vi "CRYRTA.vi"(0 "Device In":u16, 2 "Manual":bool=TRUE, 5 "Signal Path":i32(ring) caption="信号通道", 7 "Avg. Time(sec)":dbl=0.05 caption="平均时间(秒)" min=0.05 format="%.0p", 9 "Weighting":i32(ring) caption="加权" items=["Linear", "A-weighting", "B-weighting", "C-weighting", "ITU-R 468-4", "Dolby", "CCITT", "C-message", "Wb", "Wc", "Wd", "We", "Wf", "Wh", "Wj", "Wk", "Wm", "AES17 20 kHz lowpass", "AES17 40 kHz lowpass", "AES17 20 kHz highpass", "AES17 40 kHz highpass"], 11 "Start":bool, 12 "Hardware in":string, 13 "Execution control":T8={"interactive"=TRUE, "displayed"=TRUE, "in a seq"=FALSE}, 14 "Calibration in":string) -> (3 "Canceled?":bool, 4 "band power":dbl[](array[numeric]), 6 "Data output":T4, 8 "df Array":dbl[](array[numeric]), 10 "Data Out":T6={"Name"="", "Curve"=[], "X data"=1, "Y data"=1, "Z data"=1, "X axis"=0, "Y axis"=1, "Z axis"=1, "X unit"="", "Y unit"="", "Z unit"="", "X dB ref"=1.0, "Y dB ref"=1.0, "Z dB ref"=1.0, "single val"=FALSE, "protected"=FALSE, "display X"=TRUE, "display Y"=FALSE, "display Z"=TRUE, "Test Info"="", "Step No."=0, "Plot Settings"={"Color"=0, "Interpolation"=0, "Point Style"=0, "Line Style"=0, "Point Color"=0, "Line Width"=0, "Bar Plot Style"=0, "Fill To"=0}, "AutoProtect"=FALSE} {"Z data" items=["dB", "Lin"]; "X data" items=["dB", "Lin"]; "Y data" items=["dB", "Lin"]; "Z dB ref" format="%.1f"; "Z axis" items=["Log", "Lin"]; "X dB ref" format="%.1f"; "X axis" items=["Log", "Lin"]; "Y axis" items=["Log", "Lin"]; "Y dB ref" format="%.1f"; "Curve"."z" format="%.2f"; "Curve"."y" format="%.2f"; "Curve"."x" format="%.2f"}, 15 "RTA Setup Out":string)   [LabVIEW 2013]
uses:
  Typedef Control/CRYData Cluster.ctl
  Typedef Control/CRYData Variant Array.ctl
  <vilib>/addons/_NISVFA/_Shared subVIs/Controls/svc_Channel Info.ctl
  <vilib>/addons/_NISVFA/_Shared subVIs/Controls/svc_Engineering Units Text Ring.ctl
  <vilib>/addons/_NISVFA/_Shared subVIs/Controls/svc_Weighting Filter Text Ring.ctl
  Typedef Control/CRYHardware Channel Info.ctl
  <vilib>/addons/Sound and Vibration/svt_Calibration/SVL Scale Voltage to EU (1 Ch).vi
  <vilib>/addons/_NISVFA/_Shared subVIs/Common/svc_Set SV Channel Info.vi
  <vilib>/addons/_NISVFA/_Shared subVIs/Common/svc_Set SV Channel Info (variant).vi
  <vilib>/addons/_NISVFA/_Shared subVIs/Common/SVL Set dB Reference (variant).vi
  SubVI/CRYMisc vis settings global.vi
  Calibration/SubVI/CRYCal Global.vi
  CRYMainGlobal.vi
  Task Sequence/CRYProject Run Control Global.vi
  <vilib>/addons/Sound and Vibration/svt_Octave/SVT Fractional-octave Analysis (1 Ch).vi
  <vilib>/addons/_NISVFA/_Shared subVIs/Common/svc_Engineering Units to Unit Label.vi
  <vilib>/addons/_NISVFA/_Shared subVIs/Common/svc_Compute Scale Factor to Convert V to EU.vi
  <vilib>/addons/_NISVFA/_Shared subVIs/Common/svc_Set dB ref if Pascal.vi
  <vilib>/addons/_NISVFA/_Shared subVIs/Common/svc_Caller VI Returned in Error Source.vi
  <vilib>/addons/Sound and Vibration/svt_Octave/SoundVib_Octave.lvlib
  CRYSound.dll
  <vilib>/addons/Sound and Vibration/svt_Calibration/SoundVib_Calibration.lvlib
panel:
  out "cal factor":dbl
  in  "equal confidence level [dB]":dbl=1.0
  in  "channel info":T1={"sensor sensitivity [mV/EU]"=1000.0, "engineering units"=1, "dB reference [EU]"=1.0, "custom label"="EU", "weighting filter"=0, "pregain [dB]"=0.0} {"pregain [dB]" format="%.2f"; "weighting filter" items=["Linear", "A-weighting", "B-weighting", "C-weighting", "ITU-R 468-4", "Dolby", "CCITT", "C-message", "Wb", "Wc", "Wd", "We", "Wf", "Wh", "Wj", "Wk", "Wm", "AES17 20 kHz lowpass", "AES17 40 kHz lowpass", "AES17 20 kHz highpass", "AES17 40 kHz highpass"]; "dB reference [EU]" format="%^.1e"; "engineering units" items=["custom..."=0, "V"=1, "A"=21, "Pa"=2, "N"=20, "g"=3, "m/s^2"=4, "m/s"=5, "m"=6, "mm/s"=12, "mm"=13, "micron/s"=14, "micron"=15, "in/s^2"=7, "in/s"=8, "in"=9, "mil/s"=10, "mil"=11, "rad/s^2"=16, "rad/s"=17, "rad"=18, "deg/s^2"=26, "deg/s"=27, "deg"=28, "RPM"=22, "cycle/s^2"=23, "Hz"=24, "cycle"=25, "strain"=19]; "sensor sensitivity [mV/EU]" format="%.2f"}
  in  "dB ref. 2":dbl=20.0 format="%.2f"
  in  "Buf Cnt":i32
  in  "isMain":bool
  in  "Rcv Idx":u16
  in  "start_flg":u8
  out "Asio OCI":u32
  in  "ASIO_Inited":bool
  in  "Remain Data":i32[](array[numeric])
  in  "Device Name":string
  in  "Audio Driver":u16
  out "error out 2":errorcluster
  out "initialized array":i32[](array[numeric])
  in  "taskID":u32
  out "Load Test":bool
  out "Configure Data":string
  out "Set Configure":bool
  out "Signal Graph":bool caption="显示"
  out "Averaging":bool caption="平均"
  out "Spectrum1":bool caption="频谱"
  out "Input":bool caption="输入"
  out "Menu":bool=TRUE
  out "StateOut":bool=TRUE
  out "VI nID":i32
  out "Title nID":i32
  in  "delta_Y":dbl
  in  "delta_X":dbl format="%#.3p"
  in  "delta_str":string
  in  "Data In":T5
  in  "Cancel":bool
  in  "Save":bool
  in  "OK":bool
  out "AvgT":bool
  in  "Continue":bool
  in  "Time Weighting":i32(ring) caption="时间加权" items=["快", "慢", "自定义"]
  in  "Lin/Exp":i32(slide)
  in  "Octave Band":u16(ring) caption="倍频程" items=["1/1", "1/3", "1/6", "1/12", "1/24"]
  in  "Correct":bool caption="应用修正"
  in  "A/M/M":i32(slide)
  out "Real Time":u16(slide) caption="实时" scale=0.0..10.0
  out "Buffer":u16(slide) caption="缓冲器" scale=0.0..100.0
  out "Spectrum":T7(graph)={"nominal frequencies [Hz]"=[16.00000023841858, 20.0, 25.0, 31.500000953674316, 40.0, 50.0, 63.00000190734863, 80.0, 100.0, 125.0, 160.0000023841858, 200.0, 250.0, 315.00000953674316, 400.0, 500.0, 630.0000190734863, 800.0, 1000.0, 1250.0, 1600.000023841858, 2000.0, 2500.0, 3150.0000953674316, 4000.0, 5000.0, 6300.000190734863, 8000.0, 10000.0, 12500.0, 16000.00023841858, 20000.0, 25000.0, 31500.000953674316, 40000.0, 50000.0], "band power"=[-69.88905633271838, -74.01516494128754, -77.58719522671365, -75.73752952138173, -71.3505823520545, -71.81115871325046, -70.64913806002016, -71.74459815152325, -68.26393707572068, -69.54637847470994, -67.93028521843318, -67.11517882984813, -62.609020897016414, -59.9132266385828, -59.334469065938535, -58.93600195892711, -54.76273997651711, -40.68205149663691, -35.92796599129668, -52.708171896456896, -58.27685035662345, -61.23526661320974, -63.279755740002244, -64.8500026443712, -66.18360537650693, -67.37703351590173, -68.4921051421575, -69.5202741642352, -70.56777995681341, -71.50671705937012, -72.52145445138709, -73.39348059691609, -74.16354227965358, -74.79422393268355, -75.18526767722105, -75.16825214452263]}
  in  "分支常量\n（见即时帮助）":bool
  in  "Record delay (ms)":dbl=100.0 format="%.2f"
  out "Elapsed Time":dbl=0.1 caption="消耗时间" format="%#.3p"
  in  "close at end":bool
  out "avg count":i32 caption="Averages"
  in  "A-weights table":dbl[][](array[numeric])=[[0.00012901551291928683, 0.001463404113537998, 0.01066103097242493, 0.04899156950274862, 0.156669051402536, 0.37020550818873904, 0.689209635331696, 0.9999999947155233, 1.148185035046126, 1.118252632301628, 0.8802313561816225, 0.0, 0.0, 0.0, 0.0, 0.0, 0.0, 0.0, 0.0, 0.0, 0.0, 0.0, 0.0, 0.0, 0.0, 0.0, 0.0, 0.0, 0.0, 0.0, 0.0, 0.0, 0.0, 0.0, 0.0, 0.0, 0.0, 0.0, 0.0, 0.0, 0.0, 0.0, 0.0, 0.0, 0.0, 0.0, 0.0, 0.0, 0.0, 0.0, 0.0, 0.0, 0.0, 0.0, 0.0, 0.0, 0.0, 0.0, 0.0, 0.0, 0.0, 0.0, 0.0, 0.0, 0.0, 0.0, 0.0, 0.0, 0.0, 0.0, 0.0, 0.0, 0.0, 0.0, 0.0, 0.0, 0.0, 0.0, 0.0, 0.0, 0.0, 0.0, 0.0, 0.0, 0.0, 0.0, 0.0, 0.0, 0.0, 0.0, 0.0, 0.0, 0.0, 0.0, 0.0, 0.0, 0.0, 0.0, 0.0, 0.0, 0.0, 0.0, 0.0, 0.0, 0.0, 0.0, 0.0, 0.0, 0.0, 0.0, 0.0, 0.0, 0.0, 0.0, 0.0, 0.0, 0.0, 0.0, 0.0, 0.0, 0.0, 0.0, 0.0, 0.0, 0.0, 0.0, 0.0, 0.0, 0.0, 0.0, 0.0, 0.0, 0.0, 0.0, 0.0, 0.0, 0.0, 0.0, 0.0, 0.0, 0.0, 0.0, 0.0, 0.0, 0.0, 0.0, 0.0, 0.0, 0.0, 0.0, 0.0, 0.0, 0.0, 0.0, 0.0, 0.0, 0.0, 0.0, 0.0, 0.0, 0.0, 0.0, 0.0, 0.0, 0.0, 0.0, 0.0, 0.0, 0.0, 0.0, 0.0, 0.0, 0.0, 0.0, 0.0, 0.0, 0.0, 0.0, 0.0, 0.0, 0.0, 0.0, 0.0, 0.0, 0.0, 0.0, 0.0, 0.0, 0.0, 0.0, 0.0, 0.0, 0.0, 0.0, 0.0, 0.0, 0.0, 0.0, 0.0, 0.0, 0.0, 0.0, 0.0, 0.0, 0.0, 0.0, 0.0, 0.0, 0.0, 0.0, 0.0, 0.0, 0.0, 0.0, 0.0, 0.0, 0.0, 0.0, 0.0, 0.0, 0.0, 0.0, 0.0, 0.0, 0.0, 0.0, 0.0, 0.0, 0.0, 0.0, 0.0, 0.0, 0.0, 0.0, 0.0, 0.0, 0.0, 0.0, 0.0, 0.0, 0.0, 0.0, 0.0, 0.0, 0.0, 0.0, 0.0, 0.0, 0.0, 0.0, 0.0, 0.0, 0.0, 0.0, 0.0, 0.0, 0.0, 0.0, 0.0, 0.0, 0.0, 0.0, 0.0, 0.0, 0.0, 0.0, 0.0, 0.0, 0.0, 0.0, 0.0, 0.0, 0.0, 0.0, 0.0, 0.0], [5.399407495978195e-05, 0.00012901551291928683, 0.00030077593224389377, 0.0006779776875028787, 0.001463404113537998, 0.0030003304333084445, 0.00581621210485118, 0.01066103097242493, 0.018547914314881855, 0.030790110186524937, 0.04899156950274862, 0.0749323365877836, 0.11034238899050194, 0.156669051402536, 0.2149857926605078, 0.2860385580343268, 0.37020550818873904, 0.4671091612550431, 0.5748515933740767, 0.689209635331696, 0.8034638534410672, 0.9094994307304253, 0.9999999947155233, 1.0704410251961953, 1.1195518850512476, 1.148185035046126, 1.1575955360559005, 1.1480657780180865, 1.118252632301628, 1.0653659406851155, 0.9863557110490331, 0.8802313561816225, 0.7509021647928303, 0.6086168184785875, 0.4678834620808579, 0.0, 0.0, 0.0, 0.0, 0.0, 0.0, 0.0, 0.0, 0.0, 0.0, 0.0, 0.0, 0.0, 0.0, 0.0, 0.0, 0.0, 0.0, 0.0, 0.0, 0.0, 0.0, 0.0, 0.0, 0.0, 0.0, 0.0, 0.0, 0.0, 0.0, 0.0, 0.0, 0.0, 0.0, 0.0, 0.0, 0.0, 0.0, 0.0, 0.0, 0.0, 0.0, 0.0, 0.0, 0.0, 0.0, 0.0, 0.0, 0.0, 0.0, 0.0, 0.0, 0.0, 0.0, 0.0, 0.0, 0.0, 0.0, 0.0, 0.0, 0.0, 0.0, 0.0, 0.0, 0.0, 0.0, 0.0, 0.0, 0.0, 0.0, 0.0, 0.0, 0.0, 0.0, 0.0, 0.0, 0.0, 0.0, 0.0, 0.0, 0.0, 0.0, 0.0, 0.0, 0.0, 0.0, 0.0, 0.0, 0.0, 0.0, 0.0, 0.0, 0.0, 0.0, 0.0, 0.0, 0.0, 0.0, 0.0, 0.0, 0.0, 0.0, 0.0, 0.0, 0.0, 0.0, 0.0, 0.0, 0.0, 0.0, 0.0, 0.0, 0.0, 0.0, 0.0, 0.0, 0.0, 0.0, 0.0, 0.0, 0.0, 0.0, 0.0, 0.0, 0.0, 0.0, 0.0, 0.0, 0.0, 0.0, 0.0, 0.0, 0.0, 0.0, 0.0, 0.0, 0.0, 0.0, 0.0, 0.0, 0.0, 0.0, 0.0, 0.0, 0.0, 0.0, 0.0, 0.0, 0.0, 0.0, 0.0, 0.0, 0.0, 0.0, 0.0, 0.0, 0.0, 0.0, 0.0, 0.0, 0.0, 0.0, 0.0, 0.0, 0.0, 0.0, 0.0, 0.0, 0.0, 0.0, 0.0, 0.0, 0.0, 0.0, 0.0, 0.0, 0.0, 0.0, 0.0, 0.0, 0.0, 0.0, 0.0, 0.0, 0.0, 0.0, 0.0, 0.0, 0.0, 0.0, 0.0, 0.0, 0.0, 0.0, 0.0, 0.0, 0.0, 0.0, 0.0, 0.0, 0.0, 0.0, 0.0, 0.0, 0.0, 0.0, 0.0, 0.0, 0.0, 0.0, 0.0, 0.0, 0.0, 0.0, 0.0, 0.0, 0.0, 0.0, 0.0, 0.0, 0.0, 0.0, 0.0, 0.0, 0.0, 0.0, 0.0, 0.0, 0.0, 0.0, 0.0, 0.0, 0.0, 0.0, 0.0, 0.0, 0.0, 0.0, 0.0, 0.0, 0.0], [8.367843089077905e-05, 0.00012901551291928683, 0.000197701205238207, 0.00030077593224389377, 0.0004537558525726572, 0.0006779776875028787, 0.0010020521461877657, 0.001463404113537998, 0.0021097598133486134, 0.0030003304333084445, 0.0042071775532512646, 0.00581621210485118, 0.007928313709042484, 0.01066103097242493, 0.014149403982936655, 0.018547914314881855, 0.024030527738545613, 0.030790110186524937, 0.039036565356906174, 0.04899156950274862, 0.0608822293261807, 0.0749323365877836, 0.09135462337865059, 0.11034238899050194, 0.132065471964561, 0.156669051402536, 0.18427522223316958, 0.2149857926605078, 0.24888545563454106, 0.2860385580343268, 0.32648117357435763, 0.37020550818873904, 0.41713765756791077, 0.4671091612550431, 0.5198278741632266, 0.5748515933740767, 0.6315709380291434, 0.689209635331696, 0.7468467914771676, 0.8034638534410672, 0.8580134792451037, 0.9094994307304253, 0.9570545361539051, 0.9999999947155233, 1.037876206708114, 1.0704410251961953, 1.0976390517709886, 1.1195518850512476, 1.1363399019935716, 1.148185035046126, 1.1552411946705066, 1.1575955360559005, 1.1552417895398122, 1.1480657780180865, 1.1358434838302867, 1.118252632301628, 1.0948998942166022, 1.0653659406851155, 1.029270469199537, 0.9863557110490331, 0.9365833197371723, 0.8802313561816225, 0.817971279008174, 0.7509021647928303, 0.6805201645952638, 0.6086168184785875, 0.537116348933795, 0.4678834620808579, 0.4025421323855877, 0.3423424643096228, 0.0, 0.0, 0.0, 0.0, 0.0, 0.0, 0.0, 0.0, 0.0, 0.0, 0.0, 0.0, 0.0, 0.0, 0.0, 0.0, 0.0, 0.0, 0.0, 0.0, 0.0, 0.0, 0.0, 0.0, 0.0, 0.0, 0.0, 0.0, 0.0, 0.0, 0.0, 0.0, 0.0, 0.0, 0.0, 0.0, 0.0, 0.0, 0.0, 0.0, 0.0, 0.0, 0.0, 0.0, 0.0, 0.0, 0.0, 0.0, 0.0, 0.0, 0.0, 0.0, 0.0, 0.0, 0.0, 0.0, 0.0, 0.0, 0.0, 0.0, 0.0, 0.0, 0.0, 0.0, 0.0, 0.0, 0.0, 0.0, 0.0, 0.0, 0.0, 0.0, 0.0, 0.0, 0.0, 0.0, 0.0, 0.0, 0.0, 0.0, 0.0, 0.0, 0.0, 0.0, 0.0, 0.0, 0.0, 0.0, 0.0, 0.0, 0.0, 0.0, 0.0, 0.0, 0.0, 0.0, 0.0, 0.0, 0.0, 0.0, 0.0, 0.0, 0.0, 0.0, 0.0, 0.0, 0.0, 0.0, 0.0, 0.0, 0.0, 0.0, 0.0, 0.0, 0.0, 0.0, 0.0, 0.0, 0.0, 0.0, 0.0, 0.0, 0.0, 0.0, 0.0, 0.0, 0.0, 0.0, 0.0, 0.0, 0.0, 0.0, 0.0, 0.0, 0.0, 0.0, 0.0, 0.0, 0.0, 0.0, 0.0, 0.0, 0.0, 0.0, 0.0, 0.0, 0.0, 0.0, 0.0, 0.0, 0.0, 0.0, 0.0, 0.0, 0.0, 0.0, 0.0, 0.0, 0.0, 0.0, 0.0, 0.0, 0.0, 0.0, 0.0, 0.0, 0.0, 0.0, 0.0, 0.0, 0.0, 0.0, 0.0, 0.0, 0.0, 0.0, 0.0, 0.0, 0.0, 0.0, 0.0, 0.0, 0.0, 0.0, 0.0, 0.0, 0.0, 0.0, 0.0, 0.0, 0.0, 0.0, 0.0, 0.0, 0.0, 0.0, 0.0, 0.0, 0.0, 0.0, 0.0, 0.0, 0.0, 0.0, 0.0, 0.0], [0.00011583993672799015, 0.0001436292864864441, 0.0001778012603656263, 0.00021973037298173516, 0.00027102570238892744, 0.00033361829503177585, 0.00040977096445946406, 0.000502144096454577, 0.0006138152751182365, 0.0007483329340285107, 0.0009097805203891802, 0.0011028293999198581, 0.0013327910595308504, 0.0016055412855545807, 0.001927812596850252, 0.0023069345626637503, 0.0027510762632911817, 0.0032692688858618688, 0.0038713529606718092, 0.004568038488373186, 0.005370988330067639, 0.00629273027705919, 0.007347006248508048, 0.00854835390632337, 0.009912611944058519, 0.011456591976451115, 0.013198414872492882, 0.015157273683447927, 0.017353806608623748, 0.019809700002202314, 0.0225479344594536, 0.02559273234095689, 0.028969337225770848, 0.03270384735662038, 0.03682369003277181, 0.041356352073288104, 0.04633032448226266, 0.0517739915013481, 0.057715720365678666, 0.06418368835360372, 0.071205553788576, 0.07880761869752503, 0.08701565700936863, 0.09585398833098961, 0.10534521793242066, 0.1155107375037957, 0.12636988550983205, 0.13794127463318118, 0.15024113586437393, 0.1632848967869704, 0.17708626361505395, 0.1916580823381564, 0.20701225766866202, 0.22315890277798844, 0.24010772055060164, 0.2578667877323233, 0.2764428192438814, 0.29584026382455575, 0.31606163651838687, 0.3371061870135577, 0.358969471680208, 0.38164263344251637, 0.4051111260279011, 0.42935461190455376, 0.45434483933925407, 0.480045802431748, 0.5064120249737566, 0.5333885360941689, 0.5609098702676212, 0.588899974654465, 0.6172718811833343, 0.645928214660294, 0.6747620175445727, 0.7036576221391205, 0.7324922455974027, 0.7611377412235474, 0.7894627813504073, 0.8173355801049411, 0.8446260126445244, 0.8712088169880932, 0.8969654385440978, 0.9217868126028718, 0.9455750325204074, 0.968244851724287, 0.9897247443166602, 1.0099573438439453, 1.0288991360657103, 1.046520395336504, 1.062803589490304, 1.0777423665904693, 1.0913400059124783, 1.1036073660822594, 1.1145611766727053, 1.1242221862939086, 1.132613261770352, 1.1397577506544336, 1.145677844553015, 1.1503932504186614, 1.1539199208761386, 1.1562690686718506, 1.1574463130391774, 1.157451038046763, 1.1562759436684638, 1.1539067843584594, 1.150322297621406, 1.1454943493022558, 1.1393882831583702, 1.1319635038665108, 1.1231742995478864, 1.1129709826888627, 1.1013012895900083, 1.088111995241367, 1.0733511175313564, 1.0569701010320056, 1.0389265391733042, 1.0191870806799064, 0.997730470262017, 0.974550747178913, 0.9496603661952467, 0.9230931286197354, 0.8949067079177636, 0.8651846048496619, 0.8340373483677817, 0.8016026544948666, 0.7680445691386877, 0.7335512594217114, 0.698331973726688, 0.6626125963422228, 0.6266305292641101, 0.5906285479406586, 0.5548488734646586, 0.5195267345084167, 0.4848846671902413, 0.45112730190313854, 0.41843702837843694, 0.3869708391807511, 0.35685833235656267, 0.32820084229118146, 0.0, 0.0, 0.0, 0.0, 0.0, 0.0, 0.0, 0.0, 0.0, 0.0, 0.0, 0.0, 0.0, 0.0, 0.0, 0.0, 0.0, 0.0, 0.0, 0.0, 0.0, 0.0, 0.0, 0.0, 0.0, 0.0, 0.0, 0.0, 0.0, 0.0, 0.0, 0.0, 0.0, 0.0, 0.0, 0.0, 0.0, 0.0, 0.0, 0.0, 0.0, 0.0, 0.0, 0.0, 0.0, 0.0, 0.0, 0.0, 0.0, 0.0, 0.0, 0.0, 0.0, 0.0, 0.0, 0.0, 0.0, 0.0, 0.0, 0.0, 0.0, 0.0, 0.0, 0.0, 0.0, 0.0, 0.0, 0.0, 0.0, 0.0, 0.0, 0.0, 0.0, 0.0, 0.0, 0.0, 0.0, 0.0, 0.0, 0.0, 0.0, 0.0, 0.0, 0.0, 0.0, 0.0, 0.0, 0.0, 0.0, 0.0, 0.0, 0.0, 0.0, 0.0, 0.0, 0.0, 0.0, 0.0, 0.0, 0.0, 0.0, 0.0, 0.0, 0.0, 0.0, 0.0, 0.0, 0.0, 0.0, 0.0, 0.0, 0.0, 0.0, 0.0, 0.0, 0.0, 0.0, 0.0, 0.0, 0.0, 0.0, 0.0, 0.0, 0.0, 0.0, 0.0, 0.0, 0.0, 0.0, 0.0, 0.0, 0.0, 0.0, 0.0, 0.0, 0.0, 0.0, 0.0], [0.00012225672092004442, 0.00013613208222852408, 0.00015152474491120793, 0.0001685912876410086, 0.0001875024895038481, 0.00020843582576056678, 0.000231600552830374, 0.00025722548415758786, 0.0002855289289635239, 0.00031679864557676384, 0.000351291555925052, 0.00038933086776060633, 0.0004312412313259728, 0.0004773705720191734, 0.0005281224421433495, 0.0005839000265141396, 0.0006451505759304147, 0.0007123335832270973, 0.0007859971134389553, 0.000866645910773121, 0.0009549004497428776, 0.0010513292543200767, 0.0011566542967275037, 0.0012715141528389484, 0.0013967165383073849, 0.0015330023245622762, 0.0016812074021549841, 0.0018422112131822853, 0.0020169369229408292, 0.002206389379187185, 0.002411544976788906, 0.0026334575228018856, 0.002873311567204458, 0.0031322584502440844, 0.0034115397461828892, 0.003712396343881364, 0.004036215031988239, 0.004384385061676199, 0.004758343458501846, 0.005159634054815832, 0.005589793807700727, 0.006050469416386913, 0.0065433612041713735, 0.007070222047231289, 0.007632928844602979, 0.008233419004534538, 0.008873533185083996, 0.00955539033927408, 0.010281009230984933, 0.011052796225577463, 0.01187270896966456, 0.012743363008831776, 0.01366699245121816, 0.014646058159536054, 0.015683272134367158, 0.0167812101844285, 0.0179425965694284, 0.01917020465597061, 0.02046685148453447, 0.021835620098618818, 0.023279413126743746, 0.024801396510782236, 0.02640477439559649, 0.02809265507549275, 0.02986828396135696, 0.031735178074280654, 0.03369660843592097, 0.03575610603206134, 0.03791706000423899, 0.04018297427067933, 0.042557323239596045, 0.045043830397902114, 0.04764603225123459, 0.05036740205779583, 0.05321164137777925, 0.05618206522487317, 0.05928235272121169, 0.06251592481981894, 0.06588624155692245, 0.06939663312356692, 0.07305061571765548, 0.07685122633840107, 0.08080183533841384, 0.08490547665940859, 0.08916534232601793, 0.09358409309539154, 0.09816470562547887, 0.10290995571564931, 0.10782258540696482, 0.11290494602011446, 0.11815969877279844, 0.12358910711039657, 0.12919538657878887, 0.13498070440776755, 0.14094735871332803, 0.14709705951746882, 0.1534318252115702, 0.1599534436584327, 0.16666365105005457, 0.1735641308525213, 0.18065651205553968, 0.18794236660264302, 0.1954228488224075, 0.20309976426049073, 0.21097413413936192, 0.21904743735513924, 0.22732053679815653, 0.23579490634323713, 0.24447121008177145, 0.25335069198730464, 0.2624339378319428, 0.2717218992948057, 0.2812150110208473, 0.29091368749036084, 0.300818295476669, 0.3109289586739394, 0.3212456969717298, 0.3317680678845701, 0.3424954688176979, 0.35342726051653683, 0.36456224831783635, 0.37589912818065446, 0.3874358222212615, 0.39917053235195626, 0.41110046029221087, 0.42322254794095443, 0.43553342902289716, 0.4480290919832117, 0.4607051378203919, 0.4735563139304948, 0.4865769166873909, 0.49976088620278636, 0.5131013564759395, 0.5265906433478917, 0.5402206230026256, 0.5539824415478866, 0.5678667527067462, 0.5818630845016003, 0.5959608268220914, 0.6101482507640741, 0.6244132420797235, 0.6387431743663411, 0.6531243759784761, 0.6675431512492578, 0.681984828110557, 0.6964346451884604, 0.7108769753856254, 0.7252962751701603, 0.7396764437995997, 0.7540012690939792, 0.7682541360008401, 0.7824187847628459, 0.7964784463063086, 0.8104169066151684, 0.8242177707842303, 0.8378649460466877, 0.8513428384823369, 0.8646360689482658, 0.8777298220907991, 0.8906098926571995, 0.903262507060062, 0.9156747351307348, 0.9278342978440567, 0.9397297200516699, 0.95135040137708, 0.9626864091392484, 0.9737288650382403, 0.9844697136695407, 0.9949017719442329, 1.0050187243199702, 1.0148151758925124, 1.0242865554167355, 1.033429150251184, 1.04224003484883, 1.0507170561166, 1.0588587592465397, 1.0666643210877353, 1.0741336885979857, 1.0812672122645304, 1.0880658620139851, 1.0945310030851207, 1.1006644115514237, 1.1064682067340934, 1.1119447984102, 1.117096752748235, 1.121926910215412, 1.1264380967895842, 1.1306332756569393, 1.1345153609388736, 1.138087248716437, 1.1413517432913922, 1.144311477992279, 1.146968940391007, 1.149326392030887, 1.151385833041616, 1.153148992116711, 1.1546172793624818, 1.1557917648668372, 1.1566731579715792, 1.1572617902357767, 1.1575575860373175, 1.1575600627375238, 1.157268309791097, 1.1566809861826823, 1.1557963102839028, 1.1546120594626004, 1.1531255807721572, 1.1513337840103137, 1.1492331327382381, 1.1468197019646889, 1.144089147954264, 1.1410367512870832, 1.1376574272820792, 1.1339457453787871, 1.12989599480608, 1.1255021753330685, 1.1207580600366753, 1.1156572256264548, 1.1101931264984122, 1.104359096762575, 1.0981484975912152, 1.0915546745114033, 1.0845710970914006, 1.0771914239455795, 1.0694095368530765, 1.0612196939443284, 1.0526165564157512, 1.043595300780511, 1.034151737426516, 1.0242823482003527, 1.013984438996384, 1.0032562352816357, 0.9920969262367666, 0.9805068778182167, 0.9684876106160932, 0.9560418853809428, 0.9431739406984587, 0.9298894011042307, 0.916195507096381, 0.9021010035924382, 0.8876162845140686, 0.8727535245037558, 0.8575264706692125, 0.8419507387251066, 0.8260434011256425, 0.8098235090755798, 0.7933114948870663, 0.7765295182733128, 0.7595010509384336, 0.7422511193208406, 0.7248058786539537, 0.7071927338923645, 0.6894399072253197, 0.6715765139564523, 0.6536322871788603, 0.6356374570132688, 0.6176223709042133, 0.5996175871129596, 0.5816534295659871, 0.5637599223926398, 0.545966475519799, 0.5283019140820844, 0.5107941116895709, 0.49346988433858013, 0.47635487946037225, 0.45947334801192596, 0.44284808820321087, 0.4265005059785492, 0.41045020508592533, 0.39471507220518004, 0.37931133427592306, 0.3642535126107009, 0.34955416562801706, 0.3352243310062099, 0.32127303522717754, 0.30770776305027714]] format="%.5f"
  in  "cont loop":bool
  in  "Y Units":string="Pa"
  out "Channel In":u16
  in  "Channels":u8=2
  in  "Bits":i32=16
  in  "Sampling rate":dbl=44100.0
  in  "prefix In":string="u"
  in  "dB ref.":dbl=20.0 format="%.2f"
  in  "Sens":dbl=1.0 format="%.3f"
  in  "Freq, A, B, C wgt.":dbl[][](array[numeric])=[[8.0, 10.0, 12.5, 16.0, 20.0, 25.0, 31.5, 40.0, 50.0, 63.0, 80.0, 100.0, 125.0, 160.0, 200.0, 250.0, 315.0, 400.0, 500.0, 630.0, 800.0, 1000.0, 1250.0, 1600.0, 2000.0, 2500.0, 3150.0, 4000.0, 5000.0, 6300.0, 8000.0, 10000.0, 12500.0, 16000.0, 20000.0, 25000.0, 31500.0, 40000.0, 50000.0, 63000.0, 80000.0, 100000.0], [-77.55000305175781, -70.43000030517578, -63.58000183105469, -56.41999816894531, -50.38999938964844, -44.81999969482422, -39.529998779296875, -34.540000915527344, -30.270000457763672, -26.219999313354492, -22.399999618530273, -19.139999389648438, -16.190000534057617, -13.239999771118164, -10.850000381469727, -8.670000076293945, -6.639999866485596, -4.769999980926514, -3.25, -1.909999966621399, -0.7900000214576721, 0.0, 0.5799999833106995, 0.9900000095367432, 1.2000000476837158, 1.2699999809265137, 1.2000000476837158, 0.9599999785423279, 0.550000011920929, -0.11999999731779099, -1.149999976158142, -2.490000009536743, -4.25, -6.710000038146973, -9.350000381469727, -12.329999923706055, -15.699999809265137, -19.40999984741211, -23.020000457763672, -26.850000381469727, -30.8799991607666, -34.68000030517578], [-43.43000030517578, -38.2400016784668, -33.31999969482422, -28.280000686645508, -24.15999984741211, -20.479999542236328, -17.1299991607666, -14.100000381469727, -11.630000114440918, -9.359999656677246, -7.309999942779541, -5.650000095367432, -4.230000019073486, -2.940000057220459, -2.0399999618530273, -1.3600000143051147, -0.8500000238418579, -0.5, -0.2800000011920929, -0.12999999523162842, -0.03999999910593033, 0.0, 0.009999999776482582, -0.019999999552965164, -0.09000000357627869, -0.20999999344348907, -0.4000000059604645, -0.7300000190734863, -1.1799999475479126, -1.8899999856948853, -2.940000057220459, -4.300000190734863, -6.070000171661377, -8.529999732971191, -11.170000076293945, -14.15999984741211, -17.530000686645508, -21.239999771118164, -24.850000381469727, -28.68000030517578, -32.709999084472656, -36.5099983215332], [-17.59000015258789, -14.329999923706055, -11.34000015258789, -8.430000305175781, -6.21999979019165, -4.440000057220459, -3.0299999713897705, -1.9800000190734863, -1.2999999523162842, -0.8199999928474426, -0.5, -0.30000001192092896, -0.17000000178813934, -0.07999999821186066, -0.029999999329447746, 0.0, 0.019999999552965164, 0.029999999329447746, 0.029999999329447746, 0.029999999329447746, 0.019999999552965164, 0.0, -0.029999999329447746, -0.09000000357627869, -0.17000000178813934, -0.30000001192092896, -0.5, -0.8299999833106995, -1.2899999618530273, -1.9900000095367432, -3.049999952316284, -4.409999847412109, -6.179999828338623, -8.630000114440918, -11.279999732971191, -14.260000228881836, -17.639999389648438, -21.350000381469727, -24.950000762939453, -28.790000915527344, -32.81999969482422, -36.619998931884766]] format="%.2f"
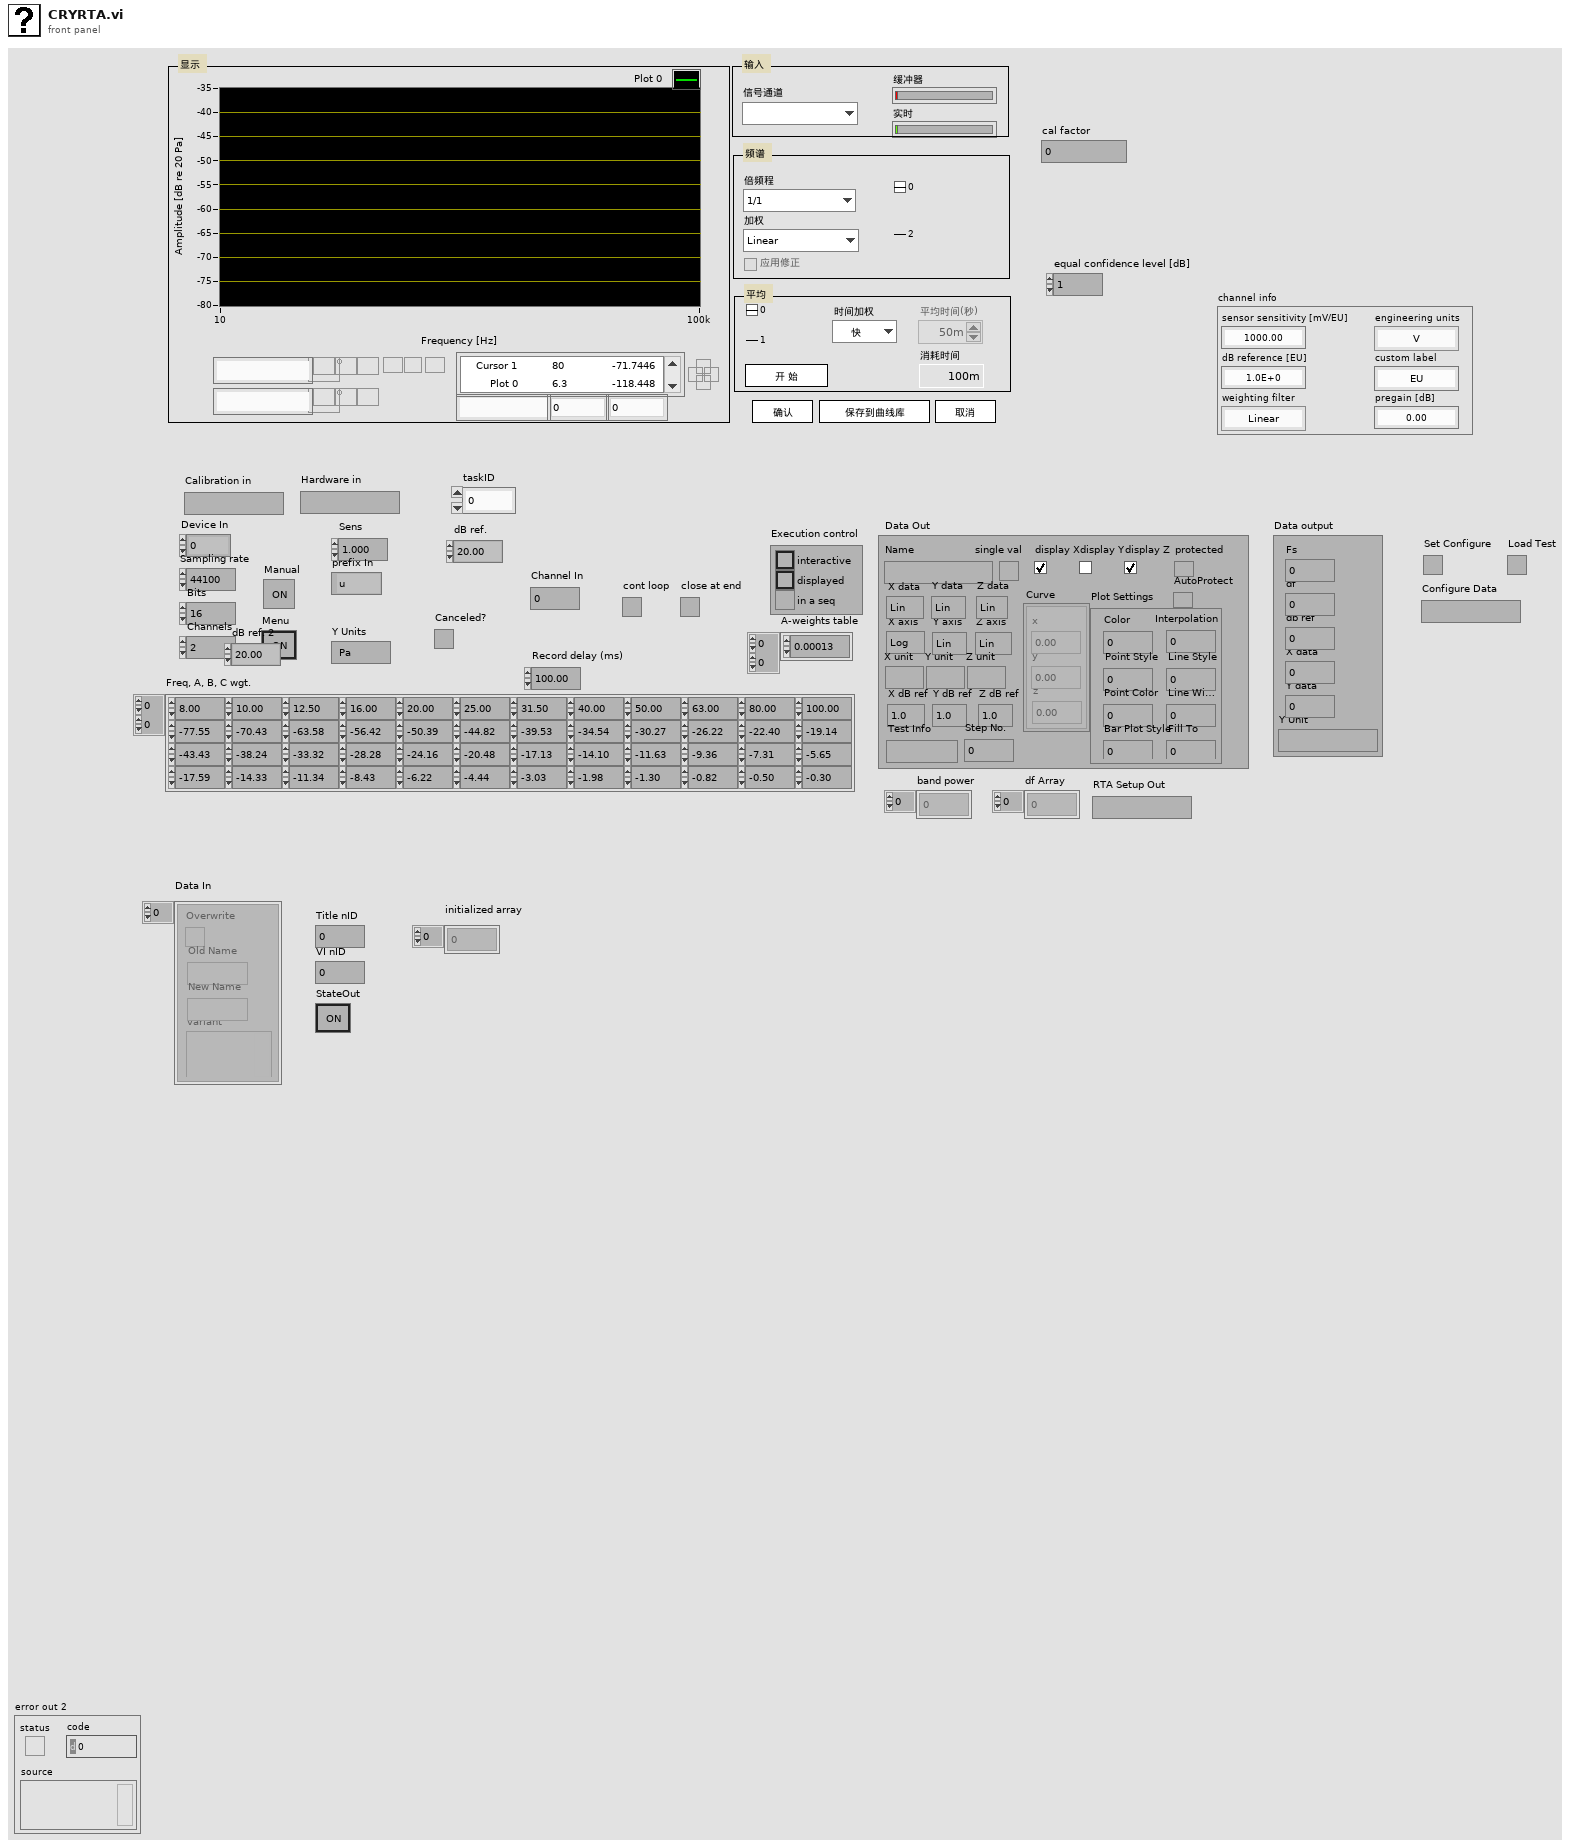
[diagram p1: front panel]
types:
  T1 = typedef "svc_Channel Info.ctl" = cluster{"sensor sensitivity [mV/EU]":dbl, "engineering units":T2, "dB reference [EU]":dbl, "custom label":string, "weighting filter":T3, "pregain [dB]":dbl}
  T2 = typedef "svc_Engineering Units Text Ring.ctl" = u16
  T3 = typedef "svc_Weighting Filter Text Ring.ctl" = u16
  T4 = cluster{"Fs":dbl, "df":dbl, "db ref":dbl, "X data":u16, "Y data":u16, "Y Unit":string}
  T5 = typedef "CRYData Variant Array.ctl" = cluster{"variant":variant, "Overwrite":bool, "Old Name":string, "New Name":string}[]
  T6 = typedef "CRYData Cluster.ctl" = cluster{"Name":string, "Curve":cluster{"x":dbl, "y":dbl, "z":dbl}[], "X data":u16, "Y data":u16, "Z data":u16, "X axis":u16, "Y axis":u16, "Z axis":u16, "X unit":string, "Y unit":string, "Z unit":string, "X dB ref":dbl, "Y dB ref":dbl, "Z dB ref":dbl, "single val":bool, "protected":bool, "display X":bool, "display Y":bool, "display Z":bool, "Test Info":string, "Step No.":i32, "Plot Settings":cluster{"Color":u32, "Interpolation":u8, "Point Style":u8, "Line Style":u8, "Point Color":u32, "Line Width":u8, "Bar Plot Style":u8, "Fill To":i16}, "AutoProtect":bool}
  T7 = cluster{"nominal frequencies [Hz]":dbl[], "band power":dbl[]}
  T8 = cluster{"interactive":bool, "displayed":bool, "in a seq":bool}
  T9 = cluster{"Octave Band":i32, "Input Channel":i32, "Time Weighting":i32, "Avg. Time(sec)":dbl, "Weighting":i32, "Lin/Exp":i32}
  T10 = enum32{"Invalid", "Default", "Floating", "Floating/Auto-Hide", "Modal"}
  T11 = cluster{"octave":i32, "det time":i32, "det sec":dbl, "lin/exp":i32, "weighting":i32, "channel":i32, "Ave/Max/Min":u16, "continuous":bool, "Applay Correction":bool, "Display":u16, "Signal Type":string}
  T12 = typedef "CRYCalibration 2DCluster.ctl" = cluster{"Calibration":T13, "Corr Curve":T6, "EQ Curve":T6, "Sens Curve":T6}
  T13 = typedef "CRYCalibration Cluster.ctl" = cluster{"Calibration Step Name":string, "Device":string, "Correction Curve Name":string, "Equalization Curve Name":string, "Sensitivity Curve Name":string, "Corr Folder and File":string, "EQ Folder and File":string, "Sens Folder and File":string, "Corr Step size":u16, "EQ Step size":u16, "Input":bool, "Last Cal Date (sec)":timestamp, "Cha Name":string, "Corr Curve Found":bool, "EQ Curve Found":bool, "Sens Curve Found":bool, "Signal Type":string, "Calibrated Device":string, "Hz":u32}
  T14 = typedef "CRYCalibration All Cluster.ctl" = cluster{"Calibration 2D":T12[], "Help":string, "Tab Value":i32, "Input Signal Type":string, "Output Signal Type":string}
  T15 = typedef "CRYHardware Channel Info.ctl" = cluster{"ID":i32, "Name":string, "Digital":bool, "Input":bool, "Device Name":string, "Hardware Ch ID":u8, "Vmax (V)":dbl, "Latency (samples)":dbl, "Sampling Rate (Hz)":u32, "Bit Depth":u32, "Anti-aliasing Factor (%fs)":sgl, "DAQmx Channel":tag, "term config":i32, "Coupling":i32, "IEPE en":bool, "ASIOChannel Name":string, "Audio Driver":u16, "ASIOChannel Index":u8}
  T16 = cluster{"acquire":bool, "FilterWidth":i32, "db-pr factor":dbl, "max level":dbl, "reset cfs":bool, "weights":dbl[], "halt acq":bool, "reset throw":bool, "cal factor":dbl, "ch left":bool, "det time":dbl, "avg type":i32, "n averaged":i32, "halt by cin":bool, "ref time":u32, "init time":u32, "start state":i32, "new weight":bool, "db weights":dbl[], "tf previous":timestamp}
  T17 = cluster{" mode":enum16{"Slow", "Fast", "Impulse", "Custom"}, "time constant [ms]":dbl}
  T18 = cluster{"low frequency":dbl, "high frequency":dbl}
  T19 = enum16{"Linear", "Exponential", "Equal confidence", "Peak"}
  T20 = cluster{"Octave Band":u16, "Signal Path":i32, "Time Weighting":i32, "Avg. Time(sec)":dbl, "Weighting":i32, "Lin/Exp":i32}
  T21 = typedef "LVCursorListTypeDef.ctl" = cluster{"Name":string, "Color":u32, "Style":u8, "Point Style":u8, "Name Visible":bool, "Allow Drag":bool, "Cursor Mode":u32, "Plot":i32, "Index":i32, "Position":cluster{"X":dbl, "Y":dbl}, "X Scale":u32, "Y Scale":u32, "Watch Plots":i32[], "Watch All Plots":bool, "Plot Area":i32, "Label Offset":cluster{"X":dbl, "Y":dbl}}[]
  T22 = cluster{"Name":string, "Color":u32, "Style":u8, "Point Style":u8, "Name Visible":bool, "Allow Drag":bool, "Cursor Mode":u32, "Plot":i32, "Index":i32, "Position":cluster{"X":dbl, "Y":dbl}, "X Scale":u32, "Y Scale":u32, "Watch Plots":i32[], "Watch All Plots":bool, "Plot Area":i32, "Label Offset":cluster{"X":dbl, "Y":dbl}}
  T23 = cluster{"Rcv Idx":i32, "Chn Idx":i32, "Data":i32[], "bufCount":i32}[]
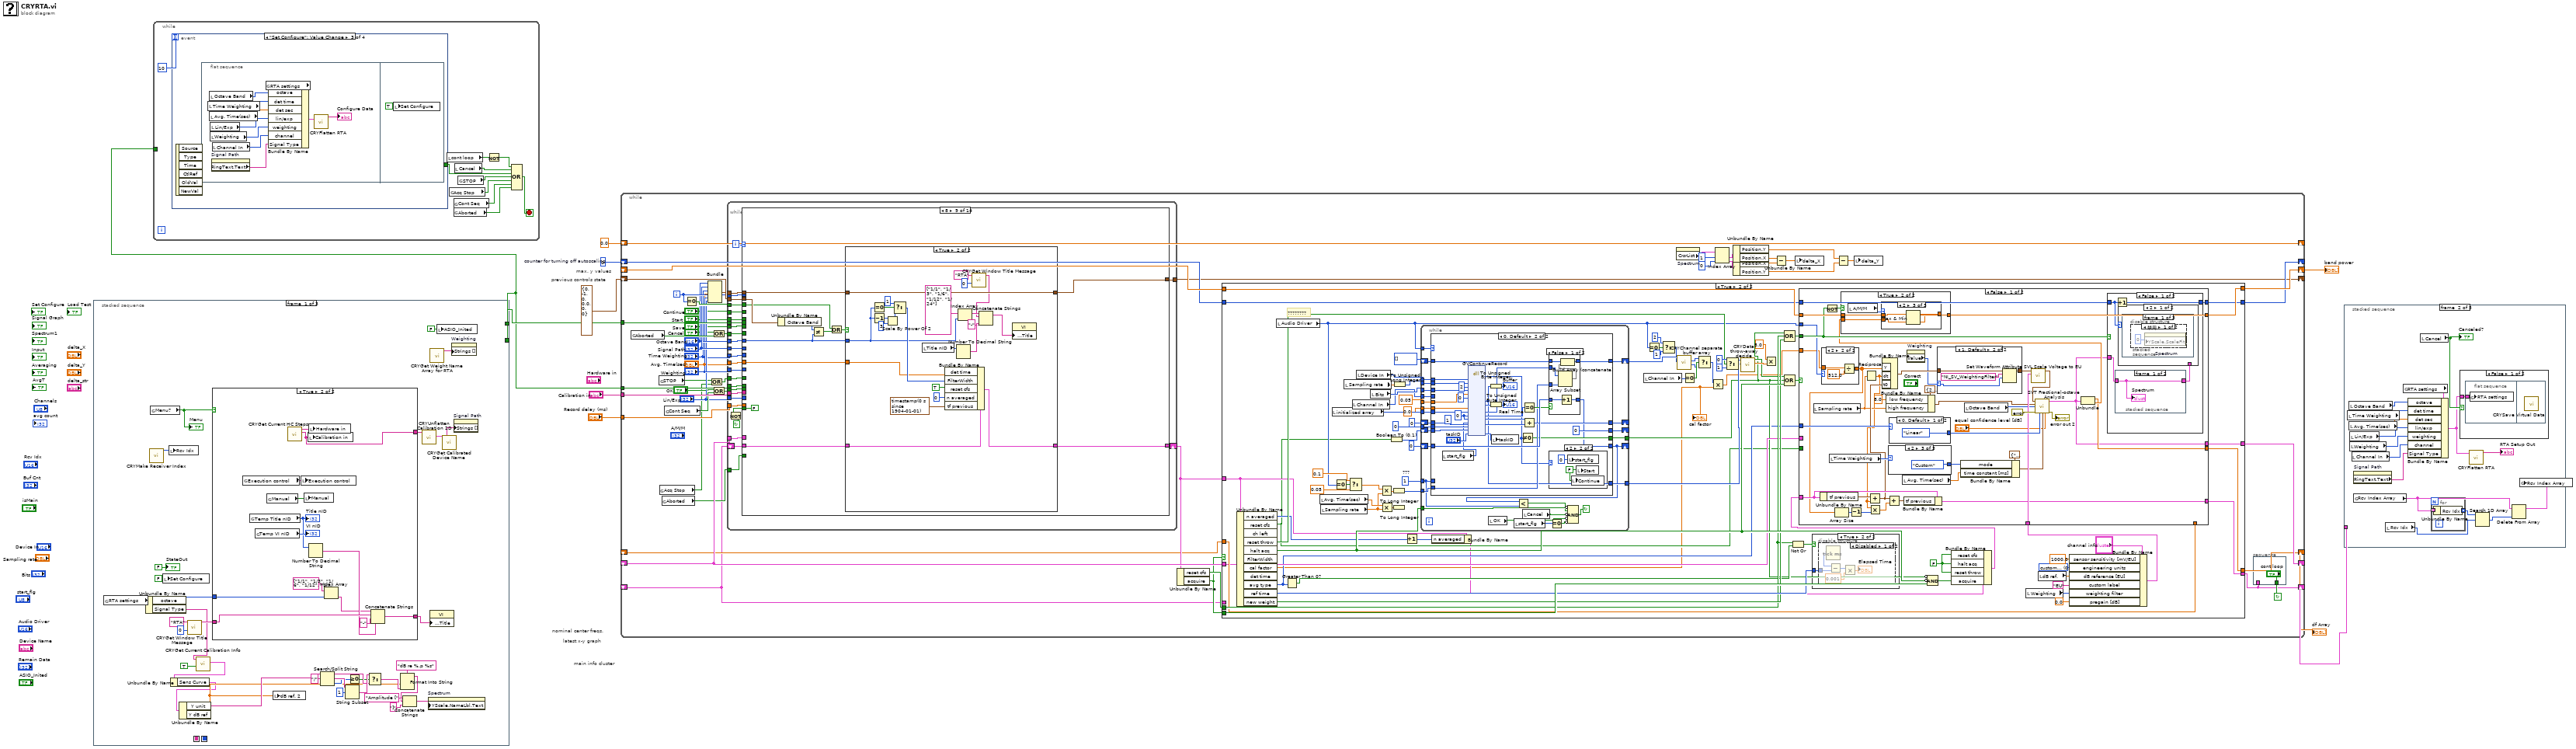
[diagram p0: block diagram]
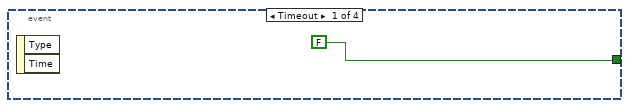
[diagram p2: hidden frame]
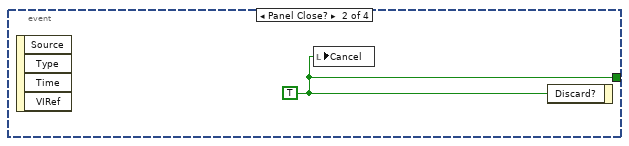
[diagram p3: hidden frame]
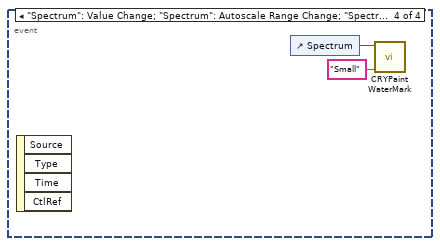
[diagram p4: hidden frame]
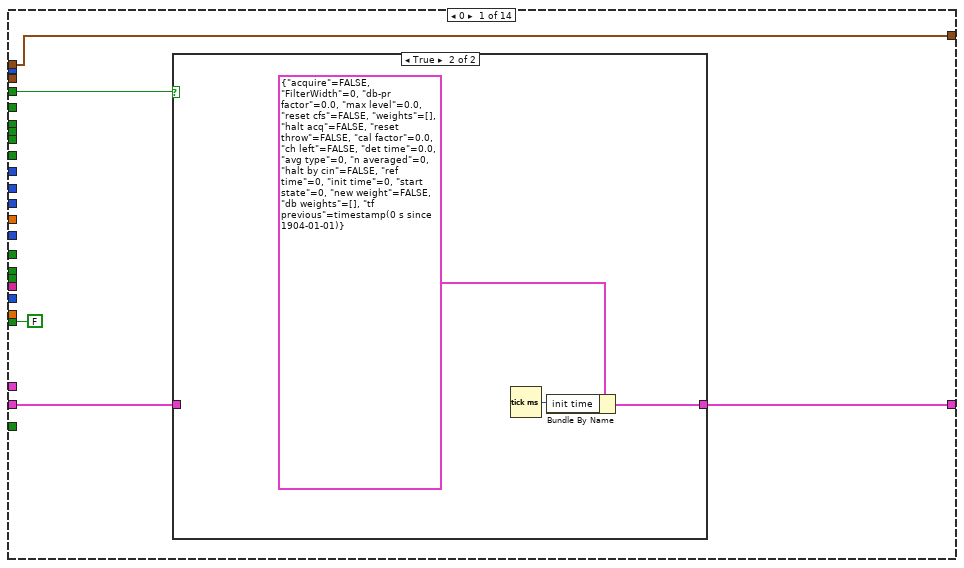
[diagram p5: hidden frame]
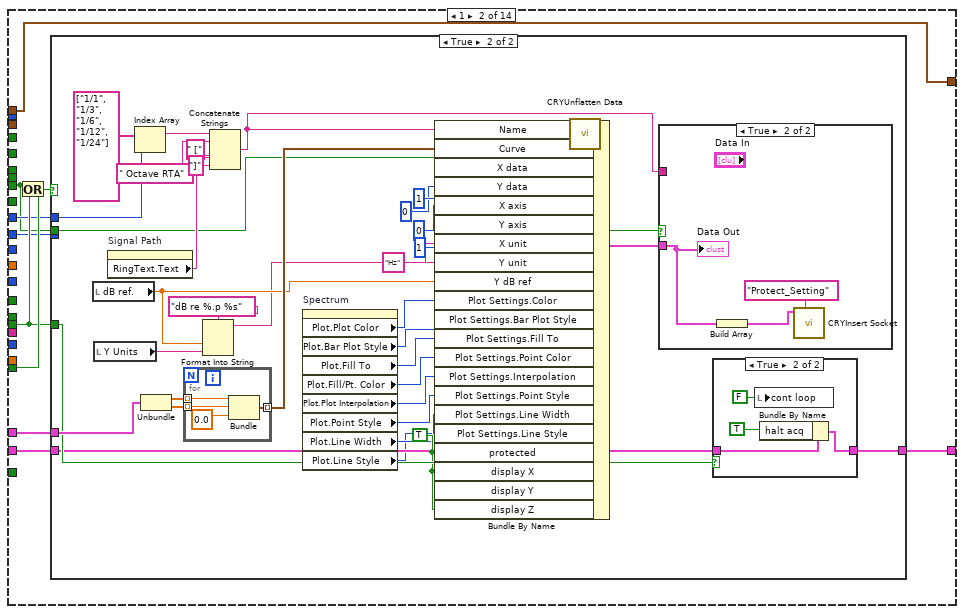
[diagram p7: hidden frame]
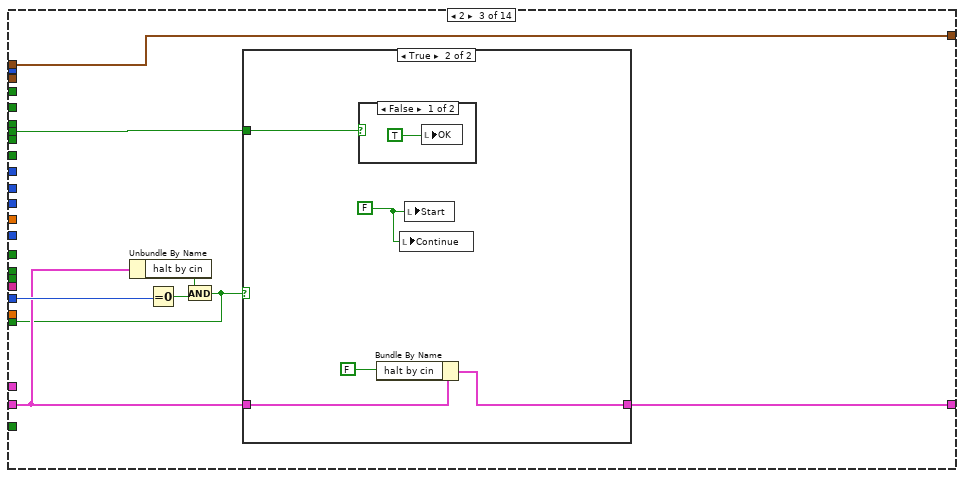
[diagram p11: hidden frame]
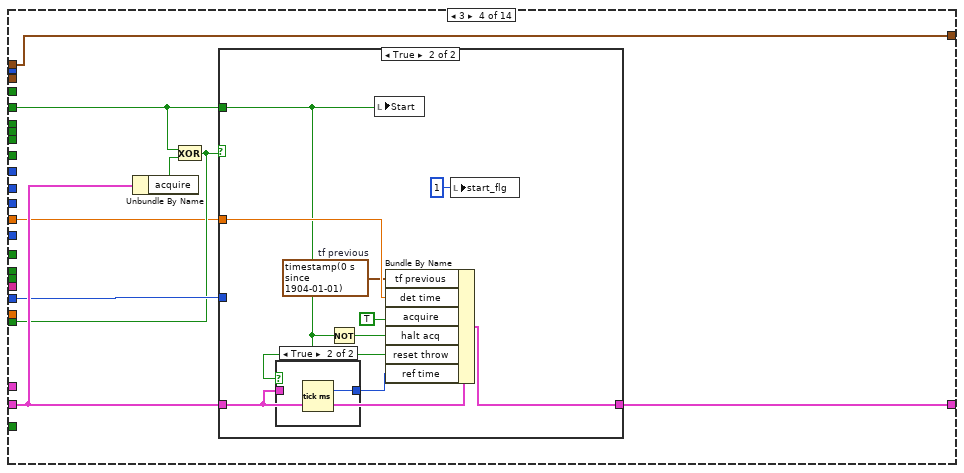
[diagram p14: hidden frame]
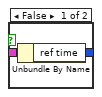
[diagram p16: hidden frame]
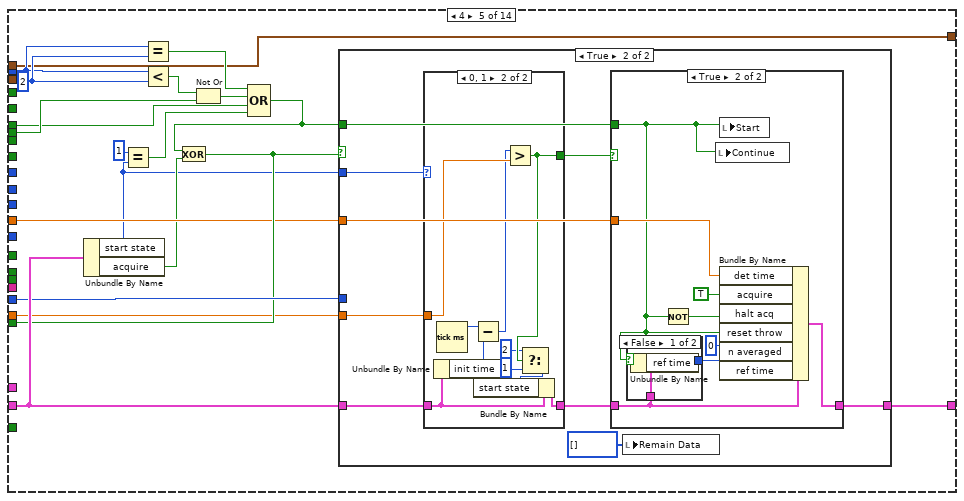
[diagram p17: hidden frame]
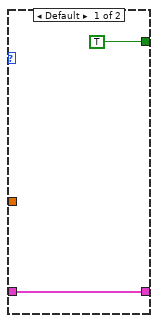
[diagram p19: hidden frame]
diagram:
  w7 = 0  # counter for turning off autoscaling
  # "max. y values"
  # "previous controls state"
  # "main info cluster"
  # "latest x-y graph"
  # "nominal center freqs."
  n1 = stacked-sequence {
    seq-local: [_ w63 _] -> [_ _ w92]
    seq-local: [_ w62 _] -> [_ _ _]
    tunnel: [_ _ "Manual"] -> w1
    tunnel: [_ w71 _] -> w8
    frame #0 {
      n2 = global read "CRYMisc vis settings global.vi" "RTA settings"() -> (w13:T11)
      n3 = Unbundle By Name(w13) -> ("octave"=w12:i32, "Signal Type"=w11:string)
      n4 = call "CRYMake Receiver Index.vi"() -> ("Receiver_Index"=w36:i32)  [unwired: 11 in]
      n5 = global read "CRYMisc vis settings global.vi" "Menu?"() -> (w43:bool)
      "Menu" <- w43
      n6 = local write "Set Configure"(FALSE ("Get Configure")) -> ()
      n7 = local write "Rcv Idx"(w36) -> ()
      n8 = call "CRYGet Window Title Message.vi"("No"=0 ("Error No"), "Kind"="RTA") -> ("Multibyte String"=w33:string)  [unwired: 4 in, 5 out]
      n9 = call "CRYGet Current Calibration Info.vi"("Is Input?"=TRUE, "Signal Type Name"=w11) -> ("Calibration All Cluster"=w14:T12)  [unwired: 9 out]
      n10 = Unbundle By Name(w14) -> ("Sens Curve"=w15:T6)
      n11 = Unbundle By Name(w15) -> ("Y unit"=w18:string, "Y dB ref"=w17:dbl)
      n12 = case shown="True" w43 {
        tunnel: [w47 w56] -> w38
        tunnel: w33 -> [w45 w55]
        tunnel: [w45 w49] -> w32
        tunnel: w12 -> [_ w48]
        frame False {
          n13 = control-ref of="This VI"() -> (w46:refnum<vi>)
          n14 = call "CRYSet RTA Front Panel.vi"("Vi Ref in"=w46) -> ()  [unwired: 10 in, 1 out]
          n15 = local read "Calibration in"() -> (w47:string)
        }
        frame True {
          n16 = global read "CRYMisc vis settings global.vi" "Execution control"() -> (w60:T8)
          n17 = global read "CRYMisc vis settings global.vi" "Temp Title nID"() -> (w53:i32)
          "Title nID" <- w53
          n18 = global read "CRYMisc vis settings global.vi" "Temp VI nID"() -> (→"VI nID":i32)
          n19 = global read "CRYMisc vis settings global.vi" "Manual"() -> (w59:bool)
          n20 = call "CRYGet Current HC Steps.vi"() -> ("Calibration setup flattened Out"=w56:string, "Hardware setup flattened Out"=w57:string)  [unwired: 10 out]
          n21 = local write "Execution control"(w60) -> ()
          n22 = local write "Manual"(w59) -> ()
          n23 = local write "Calibration in"(w56) -> ()
          n24 = local write "Hardware in"(w57) -> ()
          n25 = Number To Decimal String(number=w53) -> (decimal integer string=w52:string)  [unwired: 1 in]
          n26 = Index Array(array=string[] ["1/1", "1/3", "1/6", "1/12", "1/24"], index=w48) -> (element=w50:string)
          n27 = Concatenate Strings(w50, w55, "-" ("string"), w52) -> (w49:string)
        }
      }
      n28 = local write "dB ref. 2"(w17) -> ()
      n29 = Search/Split String(string=w18, search string/char (-)="/" ("search char (-)")) -> (substring before match=w23:string, match + rest of string=w25:string, offset of match=w21:i32)  [unwired: 1 out]
      n30 = String Subset(string=w25, offset (0)=1) -> (substring=w26:string)  [unwired: 1 in]
      n31 = Greater Or Equal To 0?(x=w21) -> (x >= 0?=w22:bool)
      n32 = Select(t=w26, s=w22, f=w23) -> (s? t:f=w19:string)
      n33 = Format Into String(format string="dB re %.p %s", w17, w19) -> (resulting string=w27:string)  [unwired: 2 in, 1 out]
      n34 = Concatenate Strings("Amplitude [" ("string"), w27, "]" ("string")) -> (w31:string)
      n35 = call "CRYUnflatten Calibration 2D.vi"("Flattened Calibration"=w38) -> ("Calibration Step Out"=w39:T14)  [unwired: 8 in, 2 out]
      n36 = property on="Spectrum" class="XYGraph (strict)"("YScale.NameLbl.Text"=w31) -> ()  [unwired: 2 in, 2 out]
      n37 = property class="VI"("Front Panel.Title"=w32) -> ()  [unwired: 2 in, 2 out]
      n38 = call "CRYGet Weight Name Array for RTA.vi"() -> ("Weighting Names"=w42:string[])  [unwired: 11 in]
      n39 = local write "ASIO_Inited"(FALSE ("ASIO_Inited")) -> ()
      n40 = call "CRYGet Calibrated Device Name.vi"("Calibration"=w39) -> ("I_Signal Type Out"=w40:string[])  [unwired: 7 in, 7 out]
      n41 = property on="Weighting" class="Ring (strict)"("Strings []"=w42) -> ()  [unwired: 2 in, 2 out]
      n42 = property on="Signal Path" class="Ring (strict)"("Strings []"=w40) -> ()  [unwired: 2 in, 2 out]
      "StateOut" <- FALSE ("StateOut")
    }
    frame #1 {
      n43 = global read "CRYMisc vis settings global.vi" "RTA settings"() -> (w61:T11)
      n44 = Unbundle By Name(w61) -> ("octave"=w70:i32, "det time"=w68:i32, "det sec"=w67:dbl, "lin/exp"=w69:i32, "weighting"=w66:i32, "channel"=w62:i32, "Signal Type"=w63:string)
      n45 = Unbundle By Name("Execution control") -> ("in a seq"=w72:bool, "interactive"=w73:bool, "displayed"=w77:bool)
      n46 = property class="VI"() -> ("前面板窗口:打开"=w76:bool)  [unwired: 2 in, 2 out]
      n47 = control-ref of="This VI"() -> (w65:refnum<vi>)
      n48 = Not(x=w72) -> (.not. x?=w71:bool)
      n49 = local write "Time Weighting"(w68) -> ()
      n50 = local write "Octave Band"(w70) -> ()
      n51 = local write "Avg. Time(sec)"(w67) -> ()
      n52 = local write "Weighting"(w66) -> ()
      n53 = local write "Lin/Exp"(w69) -> ()
      n54 = Or(x=w73, y=w77) -> (x .or. y?=w75:bool)
      n55 = property class="VI"(reference=w65, "FP.Behavior"=T10."Floating" ("Front Panel Window:Behavior")) -> ()  [unwired: 1 in, 2 out]
      n56 = Compound Arithmetic op=AND(w75, invert w76) -> (w74:bool)
      n57 = case shown="True" w75 {
        tunnel: w75 -> [_ w79]
        tunnel: w74 -> [_ _]
        frame False {
        }
        frame True {
          n58 = stacked-sequence {
            tunnel: w79 -> [w80 _ _]
            frame #0 {
              n59 = property class="VI"("前面板窗口:打开"=w80) -> ()  [unwired: 2 in, 2 out]
            }
            frame #1 {
              n60 = Wait (ms)(milliseconds to wait=u32 150) -> ()  [unwired: 1 out]
            }
            frame #2 {
            }
          }
        }
      }
      n61 = local write "close at end"(w74) -> ()
    }
    frame #2 {
      w96 = FALSE ("Stop")
      n62 = case shown="False" "Manual" {
        tunnel: [w117 w162] -> _
        tunnel: [w104 w161] -> w85
        tunnel: [w103 w160] -> w84
        tunnel: w92 -> [w114 _]
        frame False {
          n63 = global read "CRYCal Global.vi" "Calibrate"() -> (w109:bool)
          n64 = local read "Calibration in"() -> (w111:string)
          n65 = local read "Hardware in"() -> (w112:string)
          n66 = case shown="True" w109 {
            tunnel: w114 -> [w139 _]
            tunnel: [w142 w157] -> w113
            tunnel: w112 -> [w141 w159]
            tunnel: w111 -> [w140 w158]
            tunnel: [w136 w156] -> w110
            frame False {
              n67 = call "CRYGet Hardware Info From Signal Type.vi"("Calibration In"=w140, "Hardware In"=w141, "Signal Type"=w139, "In/Out?"=TRUE) -> ("Exist?"=w144:bool, "Channel Info Out"=w143:T15)  [unwired: 5 in, 1 out]
              n68 = property on="Signal Path" class="Ring (strict)"() -> ("Strings []"=w138:string[])  [unwired: 2 in, 2 out]
              n69 = case shown="False" w144 {
                tunnel: w143 -> [_ w152]
                tunnel: [w147 w152] -> w142
                tunnel: w141 -> [w150 _]
                tunnel: w140 -> [w149 _]
                tunnel: w139 -> [_ w151]
                tunnel: [w146 w151] -> w137
                frame False {
                  w146 = "Direct In 1" ("Signal Type")
                  n70 = call "CRYGet Hardware Info From Signal Type.vi"("Calibration In"=w149, "Hardware In"=w150, "Signal Type"=w146, "In/Out?"=TRUE) -> ("Channel Info Out"=w147:T15)  [unwired: 5 in, 2 out]
                }
                frame True {
                }
              }
              n71 = Search 1D Array(1D array=w138, element=w137) -> (index of element=w136:i32)  [unwired: 1 in]
            }
            frame True {
              n72 = global read "CRYCal Global.vi" "Signal Type In"() -> (w156:u16)
              n73 = property on="Signal Path" class="Ring (strict)"() -> ("Strings []"=w155:string[])  [unwired: 2 in, 2 out]
              n74 = Index Array(array=w155, index=w156) -> (element=w153:string)
              n75 = call "CRYGet Hardware Info From Signal Type.vi"("Calibration In"=w158, "Hardware In"=w159, "Signal Type"=w153, "In/Out?"=TRUE) -> ("Channel Info Out"=w157:T15)  [unwired: 5 in, 2 out]
            }
          }
          n76 = local read "ASIO_Inited"() -> (w108:bool)
          n77 = local write "Signal Path"(w110) -> ()
          n78 = Unbundle By Name(w113) -> ("ID"=w116:i32, "Sampling Rate (Hz)"=w115:u32, "Bit Depth"=w103:u32, "Hardware Ch ID"=w105:u8, "Audio Driver"=w107:u16, "Device Name"=w106:string)  [unwired: 1 out]
          "Channel In" <- w105
          n79 = To Double Precision Float(number=w115) -> (double precision float=w104:dbl)
          n80 = case shown="2" w107 {
            tunnel: w108 -> [w125 _]
            tunnel: w106 -> [w124 _]
            tunnel: w105 -> [w121 _]
            tunnel: w104 -> [w123 _]
            tunnel: w103 -> [w122 _]
            frame 2 {
              n81 = local read "Rcv Idx"() -> (w120:u16)
              n82 = case shown="False" w125 {
                tunnel: w124 -> [w133 _]
                tunnel: w121 -> [w132 _]
                tunnel: w123 -> [w131 _]
                tunnel: w122 -> [w130 _]
                frame False {
                  n83 = call "CRYASIO In & Init & Start.vi"("Bit Depth"=w130, "Sampling Rate"=w131, "Channel Index"=w132, "Device Name"=w133) -> ("bResult"=w128:bool, "ASIO Opend Channel Index"=→"Asio OCI":u32)  [unwired: 6 in]
                  n84 = local write "ASIO_Inited"(w128) -> ()
                }
                frame True {
                }
              }
              n85 = flat-sequence {
                tunnel: w121 -> [w127]
                tunnel: w120 -> [w126]
                tunnel: [w126] -> w119
                frame #0 {
                  n86 = call "CRYUpdate Receiver Index.vi"("Chn Idx"=w127, "Receiver_Index"=w126) -> ()  [unwired: 9 in]
                }
              }
              n87 = call "CRYSet Main Receiver Array.vi"("Rcv Idx"=w119) -> ("Is Main?"=w118:bool)  [unwired: 10 in]
              n88 = local write "isMain"(w118) -> ()
            }
            frame 0, Default {
              n89 = local read "Rcv Idx"() -> (w134:u16)
              n90 = call "CRYUpdate Receiver Index.vi"("Chn Idx"=-1, "Receiver_Index"=w134) -> ()  [unwired: 9 in]
            }
          }
          n91 = To Unsigned Word Integer(number=w116) -> (unsigned 16bit integer=w117:u16)
          n92 = local write "Device Name"(w106) -> ()
          n93 = local write "Audio Driver"(w107) -> ()
          n94 = local write "Bits"(w103) -> ()
          n95 = local write "Sampling rate"(w104) -> ()
          n96 = local write "Device In"(w117) -> ()
        }
        frame True {
          (unwired) T15[] [{"ID"=2, "Name"="Left", "Digital"=FALSE, "Input"=TRUE, "Device Name"="Card", "Hardware Ch ID"=0, "Vmax (V)"=10.0, "Latency (samples)"=67.0, "Sampling Rate (Hz)"=44100, "Bit Depth"=16, "Anti-aliasing Factor (%fs)"=44100.0, "DAQmx Channel"="", "term config"=0, "Coupling"=0, "IEPE en"=FALSE, "ASIOChannel Name"="", "Audio Driver"=0, "ASIOChannel Index"=0}, {"ID"=2, "Name"="Right", "Digital"=FALSE, "Input"=TRUE, "Device Name"="Card", "Hardware Ch ID"=1, "Vmax (V)"=10.0, "Latency (samples)"=67.0, "Sampling Rate (Hz)"=44100, "Bit Depth"=16, "Anti-aliasing Factor (%fs)"=44100.0, "DAQmx Channel"="", "term config"=0, "Coupling"=0, "IEPE en"=FALSE, "ASIOChannel Name"="", "Audio Driver"=0, "ASIOChannel Index"=0}] ("I_channel Info Out")
          w161 = 44100.0 ("Sampling rate")
          w160 = 16 ("Bits")
          w162 = u16 0 ("Device In")
          n97 = local write "Sampling rate"(w161) -> ()
          n98 = local write "Device In"(w162) -> ()
          n99 = local write "Bits"(w160) -> ()
          n100 = global write "CRYMainGlobal.vi" "STOP"(FALSE ("STOP")) -> ()
        }
      }
      n101 = local write "start_flg"(u8 1 ("start_flg")) -> ()
      n102 = local write "Load Test"(TRUE ("Load Test")) -> ()
      n103 = local write "delta_str"("Delta" ("delta_str")) -> ()
      n104 = local write "cont loop"(TRUE ("cont loop")) -> ()
      n105 = local write "Continue"(w96) -> ()
      n106 = local write "Cancel"(w96) -> ()
      n107 = local write "OK"(w96) -> ()
      n108 = local write "AvgT"(w96) -> ()
      n109 = local write "Start"(w96) -> ()
      n110 = stacked-sequence {
        tunnel: FALSE -> [_ w102]
        frame #0 {
          n111 = local write "avg count"(0 ("avg count")) -> ()
        }
        frame #1 {
          n112 = property on="avg count" class="DigNum (strict)"("可见"=w102) -> ()  [unwired: 2 in, 2 out]
        }
      }
      n113 = local write "Elapsed Time"(0.0 ("elapsed:")) -> ()
      n114 = property on="Spectrum" class="XYGraph (strict)"("YScale.ScaleFit"=u8 2 ("Write Attribute")) -> ()  [unwired: 2 in, 2 out]
      n115 = property on="Lin/Exp" class="Slide (strict)"("Disabled"=u8 0 ("Write Attribute")) -> ()  [unwired: 2 in, 2 out]
      n116 = To Double Precision Float(number=w85) -> (double precision float=w86:dbl)
      n117 = To Long Integer(number=w84) -> (32bit integer=w87:i32)
      n118 = Bundle(w86, "32bit integer"=2, w87) -> (w89:cluster{dbl, "32bit integer":i32, i32})  [unwired: 1 in]
      n119 = call "CRYGet Initialized WFM Array.vi"("Sound Format"=w89, "Time(s)"=0.05) -> ("initialized array"=→"initialized array":i32[])  [unwired: 8 in, 5 out]
    }
  }
  n120 = while {
    tunnel: w1 -> [_]
    stop <- w170 stop-if-true
    n121 = event shown="[2] \"Set Configure\": Value Change" {
      selector: _ -> [_ _ _ _]
      dyn-events: _ -> [_ _ _ _]
      timeout: 10 -> [_ _ _ _]
      tunnel: [FALSE ("Discard?") w175 _ _] -> w172
      event Timeout {
        n122 = event-data() -> ()  [unwired: 3 out]
      }
      event Panel Close? {
        w175 = TRUE ("Discard?")
        n123 = event-data() -> ()  [unwired: 5 out]
        n124 = local write "Cancel"(w175) -> ()
        n125 = event-data("Discard?"=w175) -> ()  [unwired: 1 in, 1 out]
      }
      event "Set Configure": Value Change {
        n126 = event-data() -> ()  [unwired: 7 out]
        n127 = flat-sequence {
          frame #0 {
            n128 = local read "Time Weighting"() -> (w183:i32)
            n129 = local read "Octave Band"() -> (w184:u16)
            n130 = local read "Avg. Time(sec)"() -> (w182:dbl)
            n131 = local read "Weighting"() -> (w180:i32)
            n132 = local read "Lin/Exp"() -> (w181:i32)
            n133 = property on="Signal Path" class="Ring (strict)"() -> ("RingText.Text"=w178:string)  [unwired: 2 in, 2 out]
            n134 = local read "Channel In"() -> (w179:u16)
            n135 = global read "CRYMisc vis settings global.vi" "RTA settings"() -> (w176:T11)
            n136 = Bundle By Name(cluster=w176, "octave"=w184, "det time"=w183, "det sec"=w182, "lin/exp"=w181, "weighting"=w180, "channel"=w179, "Signal Type"=w178) -> (w185:T11)
            n137 = call "CRYFlatten RTA.vi"("RTA settings"=w185) -> ("Flat RTA settings"=→"Configure Data":string)  [unwired: 10 out]
          }
          frame #1 {
            n138 = local write "Set Configure"(TRUE ("Get Configure")) -> ()
          }
        }
      }
      event "Spectrum": Value Change; "Spectrum": Autoscale Range Change; "Spectrum": Plot Attribute Change; "Spectrum": Scale Range Change {
        n139 = event-data() -> ()  [unwired: 5 out]
        n140 = control-ref of="Spectrum"() -> (w188:refnum<vi>)
        n141 = call "CRYPaint WaterMark.vi"("Type"="Small", "Graph Ref"=w188) -> ()  [unwired: 10 in]
      }
    }
    n142 = local read "cont loop"() -> (w168:bool)
    n143 = global read "CRYMainGlobal.vi" "Acq Stop"() -> (w166:bool)
    n144 = global read "CRYProject Run Control Global.vi" "Cont Seq"() -> (w165:bool)
    n145 = global read "CRYProject Run Control Global.vi" "Aborted"() -> (w164:bool)
    n146 = local read "Cancel"() -> (w171:bool)
    n147 = global read "CRYMainGlobal.vi" "STOP"() -> (w169:bool)
    n148 = Not(x=w168) -> (.not. x?=w167:bool)
    n149 = Compound Arithmetic op=OR(w167, w171, w172, w169, w166, w165, w164) -> (w170:bool)
  }
  n150 = while {
    tunnel: "Record delay (ms)" -> [w221]
    shift-left: w7 -> [w223]
    shift-right: [w222] -> _
    tunnel: w8 -> [w230]
    shift-left: _ -> [w235]
    shift-right: [w234] -> w5
    shift-left: T9 {"Octave Band"=0, "Input Channel"=-1, "Time Weighting"=0, "Avg. Time(sec)"=0.0, "Weighting"=0, "Lin/Exp"=0} -> [w236]
    shift-right: [w208] -> _
    shift-left: _ -> [w237]
    shift-right: [w238] -> _
    tunnel: "Calibration in" -> [w240]
    tunnel: w1 -> [w241]
    shift-left: _ -> [w189]
    shift-right: [w232] -> w9
    shift-right: [w203] -> _
    shift-left: 0.0 ("delta_Y") -> [w203]
    shift-right: [w233] -> w4
    shift-left: _ -> [w191]
    i -> [w229]
    stop <- w239 continue-if-true
    n151 = global read "CRYProject Run Control Global.vi" "Aborted"() -> (w226:bool)
    n152 = global read "CRYMainGlobal.vi" "STOP"() -> (w207:bool)
    n153 = global read "CRYMainGlobal.vi" "Acq Stop"() -> (w206:bool)
    n154 = global read "CRYProject Run Control Global.vi" "Aborted"() -> (w204:bool)
    n155 = global read "CRYProject Run Control Global.vi" "Cont Seq"() -> (w228:bool)
    n156 = Equal To 0?(x=w229) -> (x = 0?=w242:bool)
    n157 = Bundle("Octave Band"="Octave Band", "Signal Path"="Signal Path", "Time Weighting"="Time Weighting", "Avg. Time(sec)"="Avg. Time(sec)", "Weighting"="Weighting", "Lin/Exp"="Lin/Exp") -> (w209:T20)  [unwired: 1 out]
    n158 = Or(x=w207, y=w206) -> (x .or. y?=w205:bool)
    n159 = Or(x="Cancel", y=w226) -> (x .or. y?=w225:bool)
    n160 = Or(x="OK", y=w228) -> (x .or. y?=w227:bool)
    n161 = while {
      tunnel: w221 -> [w247]
      tunnel: w229 -> [w248]
      tunnel: w230 -> [w249]
      tunnel: w227 -> [w250]
      tunnel: "Start" -> [w251]
      tunnel: "Lin/Exp" -> [w252]
      tunnel: w237 -> [w253]
      tunnel: w240 -> [w254]
      tunnel: w241 -> [w255]
      shift-left: w189 -> [w257]
      shift-right: [w256] -> w224
      tunnel: w242 -> [w258]
      tunnel: w205 -> [w259]
      tunnel: "Weighting" -> [w260]
      tunnel: "Avg. Time(sec)" -> [w261]
      tunnel: "Time Weighting" -> [w262]
      tunnel: "Signal Path" -> [w263]
      tunnel: "Octave Band" -> [w264]
      tunnel: w225 -> [w265]
      tunnel: "Save" -> [w266]
      tunnel: "Continue" -> [w268]
      tunnel: w236 -> [w267]
      tunnel: w209 -> [w246]
      tunnel: [w245] -> w208
      tunnel: w204 -> [w244]
      i -> [w243]
      stop <- w269 continue-if-true
      n162 = case shown="8" w243 {
        tunnel: [FALSE w287 w339 w355 w389 w429 w452 FALSE ("x .or. y?") FALSE FALSE FALSE FALSE w705 TRUE] -> w270
        tunnel: w268 -> [_ _ _ w357 _ _ _ _ _ _ _ _ _ _]
        tunnel: w267 -> [_ _ _ _ _ w437 _ _ w499 w537 w654 w681 w710 _]
        tunnel: w266 -> [_ w280 _ _ _ _ _ _ _ _ _ _ _ _]
        tunnel: w265 -> [_ _ _ _ _ _ w455 _ _ _ _ _ _ _]
        tunnel: w264 -> [_ w283 _ _ _ _ _ w473 w492 _ w646 _ _ _]
        tunnel: w263 -> [_ w282 _ _ _ _ _ _ _ w532 _ _ _ _]
        tunnel: w262 -> [_ _ _ _ _ _ _ _ _ _ _ w675 w707 _]
        tunnel: w261 -> [_ _ _ w354 w386 _ _ w472 w491 _ _ w674 w706 w726]
        tunnel: w260 -> [_ _ _ _ _ _ _ w468 _ _ w649 _ _ _]
        tunnel: w259 -> [_ _ _ _ _ _ w454 _ _ _ _ _ _ _]
        tunnel: w258 -> [w272 _ _ _ _ w431 _ _ w488 w525 w648 w679 _ _]
        tunnel: w257 -> [w274 w285 w343 w359 w391 w435 w458 w475 w494 w534 w651 w677 w708 w736]
        tunnel: [w273 w284 w342 w360 w392 w434 w457 w474 w493 w533 w650 w676 w702 w734] -> w256
        tunnel: w255 -> [_ _ _ _ _ _ _ _ _ w531 _ _ _ _]
        tunnel: w254 -> [_ _ _ _ _ _ _ _ _ w530 _ _ _ _]
        tunnel: w253 -> [_ w288 _ _ _ _ _ _ _ _ _ _ _ _]
        tunnel: w252 -> [_ _ w345 w358 w390 w433 _ _ _ _ _ _ _ w737]
        tunnel: w251 -> [_ _ _ _ w381 _ _ _ _ _ _ _ _ _]
        tunnel: w250 -> [_ w286 _ _ _ _ _ _ _ _ _ _ _ _]
        tunnel: w249 -> [_ _ w341 _ w388 _ _ _ _ _ _ _ _ w735]
        tunnel: w248 -> [_ _ _ _ w384 _ _ _ _ _ _ _ _ _]
        tunnel: w247 -> [_ _ _ _ w379 _ _ _ _ _ _ _ _ _]
        tunnel: w246 -> [w271 w281 w338 w353 w374 w428 w456 w469 w490 w526 w644 w671 w704 w738]
        tunnel: [w271 w281 w338 w353 w374 w427 w456 w469 w489 w529 w643 w670 w703 w738] -> w245
        tunnel: w244 -> [_ _ _ _ _ _ w453 _ _ _ _ _ _ _]
        frame 0 {
          n163 = case shown="True" w272 {
            tunnel: w274 -> [w276 _]
            tunnel: [w276 w277] -> w273
            frame False {
            }
            frame True {
              n164 = Tick Count (ms)() -> (millisecond timer value=w279:u32)
              n165 = Bundle By Name(cluster=T16 {"acquire"=FALSE, "FilterWidth"=0, "db-pr factor"=0.0, "max level"=0.0, "reset cfs"=FALSE, "weights"=[], "halt acq"=FALSE, "reset throw"=FALSE, "cal factor"=0.0, "ch left"=FALSE, "det time"=0.0, "avg type"=0, "n averaged"=0, "halt by cin"=FALSE, "ref time"=0, "init time"=0, "start state"=0, "new weight"=FALSE, "db weights"=[], "tf previous"=timestamp(0 s since 1904-01-01)}, "init time"=w279) -> (w277:T16)
            }
          }
        }
        frame 1 {
          n166 = Or(x=w280, y=w286) -> (x .or. y?=w287:bool)
          n167 = case shown="True" w287 {
            tunnel: w288 -> [_ w322]
            tunnel: w286 -> [_ w317]
            tunnel: w285 -> [w289 w316]
            tunnel: [w289 w315] -> w284
            tunnel: w283 -> [_ w314]
            tunnel: w282 -> [_ _]
            tunnel: w280 -> [_ w306]
            frame False {
            }
            frame True {
              w295 = TRUE ("protected")
              n168 = local read "dB ref."() -> (w300:dbl)
              n169 = local read "Y Units"() -> (w302:string)
              n170 = property on="Signal Path" class="Ring (strict)"() -> ("RingText.Text"=w307:string)  [unwired: 2 in, 2 out]
              n171 = Index Array(array=string[] ["1/1", "1/3", "1/6", "1/12", "1/24"], index=w314) -> (element=w312:string)
              n172 = Unbundle(w322) -> ("nominal frequencies [Hz]"=w321:dbl[], "band power"=w320:dbl[])
              n173 = for {
                tunnel: [w336] -> w325 mode=indexing
                tunnel: w321 -> [w335] mode=indexing
                tunnel: w320 -> [w334] mode=indexing
                n174 = Bundle(w335, w334, 0.0) -> (w336:cluster{dbl, dbl, dbl})  [unwired: 1 out]
              }
              n175 = Format Into String(format string="dB re %.p %s", w300, w302) -> (resulting string=w299:string)  [unwired: 2 in, 1 out]
              n176 = Concatenate Strings(w312, " Octave RTA", " [" ("string"), w307, "]" ("string")) -> (w305:string)
              n177 = property on="Spectrum" class="XYGraph (strict)"() -> ("Plot.Plot Color"=w298:u32, "Plot.Bar Plot Style"=w293:u8, "Plot.Fill To"=w297:i16, "Plot.Fill/Pt. Color"=w296:u32, "Plot.Plot Interpolation"=w294:u8, "Plot.Point Style"=w292:u8, "Plot.Line Width"=w291:u8, "Plot.Line Style"=w290:u8)  [unwired: 2 in, 2 out]
              n178 = call "CRYUnflatten Data.vi"() -> ("Datum"=w304:T6)  [unwired: 1 in, 10 out]
              n179 = Bundle By Name(cluster=w304, "Name"=w305, "Curve"=w325, "X data"=u16 1 ("Bundle Element"), "Y data"=u16 0 ("Bundle Element"), "X axis"=u16 0 ("Bundle Element"), "Y axis"=u16 1 ("Bundle Element"), "X unit"="Hz" ("Bundle Element"), "Y unit"=w299, "Y dB ref"=w300, "Plot Settings.Color"=w298, "Plot Settings.Bar Plot Style"=w293, "Plot Settings.Fill To"=w297, "Plot Settings.Point Color"=w296, "Plot Settings.Interpolation"=w294, "Plot Settings.Point Style"=w292, "Plot Settings.Line Width"=w291, "Plot Settings.Line Style"=w290, "protected"=w295, "display X"=w295, "display Y"=w295, "display Z"=w295) -> (w310:T6)
              n180 = case shown="True" w306 {
                tunnel: w310 -> [_ w327]
                tunnel: w305 -> [_ _]
                frame False {
                }
                frame True {
                  n181 = Build Array(w327) -> (w326:T6[])
                  n182 = call "CRYInsert Socket.vi"("sOption1"="Protect_Setting" ("sOption"), "Curves"=w326) -> ()  [unwired: 9 in, 1 out]
                  "Data Out" <- w327
                }
              }
              n183 = case shown="True" w317 {
                tunnel: w316 -> [w329 w332]
                tunnel: [w329 w331] -> w315
                frame False {
                }
                frame True {
                  n184 = local write "cont loop"(FALSE ("cont loop")) -> ()
                  n185 = Bundle By Name(cluster=w332, "halt acq"=TRUE ("Bundle Element")) -> (w331:T16)
                }
              }
            }
          }
        }
        frame 2 {
          n186 = Unbundle By Name(w343) -> ("halt by cin"=w344:bool)
          n187 = Equal To 0?(x=w345) -> (x = 0?=w340:bool)
          n188 = And(x=w344, y=w340) -> (x .and. y?=w339:bool)
          n189 = case shown="True" w339 {
            tunnel: [w346 w350] -> w342
            tunnel: w343 -> [w346 w351]
            tunnel: w341 -> [_ w349]
            frame False {
            }
            frame True {
              w347 = FALSE ("start")
              n190 = case shown="False" w349 {
                frame False {
                  n191 = local write "OK"(TRUE ("ok")) -> ()
                }
                frame True {
                }
              }
              n192 = Bundle By Name(cluster=w351, "halt by cin"=FALSE ("Bundle Element")) -> (w350:T16)
              n193 = local write "Continue"(w347) -> ()
              n194 = local write "Start"(w347) -> ()
            }
          }
        }
        frame 3 {
          n195 = Unbundle By Name(w359) -> ("acquire"=w356:bool)
          n196 = Exclusive Or(1:w356, 2:w357) -> (0:w355:bool)
          n197 = case shown="True" w355 {
            tunnel: [w361 w370] -> w360
            tunnel: w359 -> [w361 w365]
            tunnel: w357 -> [_ w364]
            tunnel: w358 -> [_ _]
            tunnel: w354 -> [_ w367]
            frame False {
            }
            frame True {
              w362 = timestamp(0 s since 1904-01-01)  # tf previous
              n198 = case shown="True" w364 {
                tunnel: [w371 w373] -> w366
                tunnel: w365 -> [w372 _]
                frame False {
                  n199 = Unbundle By Name(w372) -> ("ref time"=w371:u32)
                }
                frame True {
                  n200 = Tick Count (ms)() -> (millisecond timer value=w373:u32)
                }
              }
              n201 = Not(x=w364) -> (.not. x?=w368:bool)
              n202 = local write "Start"(w364) -> ()
              n203 = Bundle By Name(cluster=w365, "tf previous"=w362, "det time"=w367, "acquire"=TRUE ("Bundle Element"), "halt acq"=w368, "reset throw"=w364, "ref time"=w366) -> (w370:T16)
              n204 = local write "start_flg"(u8 1 ("start_flg")) -> ()
            }
          }
        }
        frame 4 {
          w385 = 2 ("y")
          n205 = Unbundle By Name(w391) -> ("start state"=w375:i32, "acquire"=w378:bool)
          n206 = Equal?(x=1 ("Output Element"), y=w375) -> (x = y?=w376:bool)
          n207 = Equal?(x=w384, y=w385) -> (x = y?=w383:bool)
          n208 = Less?(x=w384, y=w385) -> (x < y?=w387:bool)
          n209 = Not Or(1:w388, 2:w387) -> (0:w382:bool)
          n210 = Compound Arithmetic op=OR(w383, w382, w381, w376) -> (w380:bool)
          n211 = Exclusive Or(1:w378, 2:w380) -> (0:w389:bool)
          n212 = case shown="True" w389 {
            tunnel: [w393 w402] -> w392
            tunnel: w391 -> [w393 w397]
            tunnel: w380 -> [_ w400]
            tunnel: w390 -> [_ _]
            tunnel: w386 -> [_ w401]
            tunnel: w379 -> [_ w395]
            tunnel: w375 -> [_ w399]
            frame False {
            }
            frame True {
              n213 = case shown="0, 1" w399 {
                tunnel: [TRUE w408] -> w398
                tunnel: w397 -> [w403 w410]
                tunnel: [w403 w409] -> w396
                tunnel: w395 -> [_ w412]
                frame Default {
                }
                frame 0, 1 {
                  n214 = Unbundle By Name(w410) -> ("init time"=w413:u32)
                  n215 = Tick Count (ms)() -> (millisecond timer value=w414:u32)
                  n216 = Subtract(x=w414, y=w413) -> (x-y=w411:u32)
                  n217 = Greater?(x=w411, y=w412) -> (0:w408:bool)
                  n218 = Select(t=2 ("Bundle Element"), s=w408, f=1 ("Bundle Element")) -> (s? t:f=w405:i32)
                  n219 = Bundle By Name(cluster=w410, "start state"=w405) -> (w409:T16)
                }
              }
              n220 = case shown="True" w398 {
                tunnel: [w415 w423] -> w402
                tunnel: w401 -> [_ w419]
                tunnel: w396 -> [w415 w417]
                tunnel: w400 -> [_ w416]
                frame False {
                }
                frame True {
                  n221 = case shown="False" w416 {
                    tunnel: [w425 w426] -> w418
                    tunnel: w417 -> [w424 _]
                    frame False {
                      n222 = Unbundle By Name(w424) -> ("ref time"=w425:u32)
                    }
                    frame True {
                      n223 = Tick Count (ms)() -> (millisecond timer value=w426:u32)
                    }
                  }
                  n224 = Not(x=w416) -> (.not. x?=w421:bool)
                  n225 = local write "Continue"(w416) -> ()
                  n226 = local write "Start"(w416) -> ()
                  n227 = Bundle By Name(cluster=w417, "det time"=w419, "acquire"=TRUE ("Bundle Element"), "halt acq"=w421, "reset throw"=w416, "n averaged"=0 ("Bundle Element"), "ref time"=w418) -> (w423:T16)
                }
              }
              n228 = local write "Remain Data"(i32[] [] ("Remain Data")) -> ()
            }
          }
        }
        frame 5 {
          n229 = Unbundle By Name(w437) -> ("Lin/Exp"=w436:i32)
          n230 = Not Equal?(x=w436, y=w433) -> (x != y?=w430:bool)
          n231 = Or(x=w431, y=w430) -> (x .or. y?=w432:bool)
          n232 = Compound Arithmetic op=AND(w430, invert w431) -> (w429:bool)
          n233 = case shown="True" w432 {
            tunnel: w435 -> [w439 w451]
            tunnel: [w439 w450] -> w434
            tunnel: w433 -> [_ w449]
            tunnel: w428 -> [w438 w442]
            tunnel: [w438 w442] -> w427
            frame False {
            }
            frame True {
              n234 = Greater Than 0?(x=w449) -> (x > 0?=w443:bool)
              n235 = Tick Count (ms)() -> (millisecond timer value=w444:u32)
              n236 = Select(t=u8 2 ("Write Attribute"), s=w443, f=u8 0 ("Write Attribute")) -> (s? t:f=w445:u8)
              n237 = property on="Continue" class="Bool (strict)"("Visible"=w443) -> ()  [unwired: 2 in, 2 out]
              n238 = Bundle By Name(cluster=w451, "reset cfs"=TRUE, "ref time"=w444, "avg type"=w449, "n averaged"=0 ("Bundle Element")) -> (w450:T16)
              n239 = Not(x=w443) -> (.not. x?=w441:bool)
              n240 = property on="Elapsed Time" class="DigNum (strict)"("禁用"=w445) -> ()  [unwired: 2 in, 2 out]
              n241 = property on="Start" class="Bool (strict)"("Visible"=w441) -> ()  [unwired: 2 in, 2 out]
              n242 = property on="Elapsed Time" class="DigNum (strict)"("Visible"=w441) -> ()  [unwired: 2 in, 2 out]
              n243 = property on="AvgT" class="Bool (strict)"("Visible"=w443) -> ()  [unwired: 2 in, 2 out]
            }
          }
        }
        frame 6 {
          n244 = Compound Arithmetic op=OR(w455, w454, w453) -> (w452:bool)
          n245 = case shown="True" w452 {
            tunnel: w458 -> [w459 w462]
            tunnel: [w459 w461] -> w457
            frame False {
            }
            frame True {
              n246 = local write "cont loop"(FALSE ("cont loop")) -> ()
              n247 = Bundle By Name(cluster=w462, "acquire"=FALSE, "halt acq"=TRUE ("Bundle Element")) -> (w461:T16)
            }
          }
        }
        frame 7 {
          n248 = Unbundle By Name(w475) -> ("reset cfs"=w471:bool, "new weight"=w470:bool)
          n249 = local read "Sampling rate"() -> (w467:dbl)
          n250 = Or(x=w471, y=w470) -> (x .or. y?=w465:bool)
          n251 = case shown="True" w465 {
            tunnel: [w476 w483] -> w474
            tunnel: w475 -> [w476 w482]
            tunnel: w473 -> [_ w486]
            tunnel: w472 -> [_ w484]
            tunnel: w468 -> [_ w477]
            tunnel: w467 -> [_ _]
            frame False {
            }
            frame True {
              w487 = TRUE ("Bundle Element")
              w478 = FALSE ("Bundle Element")
              n252 = Less?(x=w486, y=2 ("Octave")) -> ()  [unwired: 1 out]
              n253 = local read "Freq, A, B, C wgt."() -> (w481:dbl[][])
              n254 = Unbundle By Name(w482) -> ("db weights"=w479:dbl[])
              n255 = Index Array(array=w481, index (row)=w477) -> (element=w480:dbl[])  [unwired: 1 in]
              n256 = call "CRYRta weights interpolate.vi"("Weights in dB"=w479, "Frequencies of weights array"=w480) -> ()  [unwired: 1 in, 9 out]
              n257 = Bundle By Name(cluster=w482, "reset cfs"=w478, "new weight"=w478, "acquire"=w487, "halt acq"=w487, "det time"=w484) -> (w483:T16)
            }
          }
        }
        frame 8 {
          n258 = Unbundle By Name(w499) -> ("Octave Band"=w498:i32)
          n259 = Not Equal?(x=w498, y=w492) -> (x != y?=w496:bool)
          n260 = Or(x=w488, y=w496) -> (x .or. y?=w497:bool)
          n261 = case shown="True" w497 {
            tunnel: w494 -> [w501 w512]
            tunnel: [w501 w519] -> w493
            tunnel: w492 -> [_ w515]
            tunnel: w491 -> [_ w513]
            tunnel: w490 -> [w500 w510]
            tunnel: [w500 w510] -> w489
            frame False {
            }
            frame True {
              n262 = Equal To 0?(x=w515) -> (x = 0?=w521:bool)
              n263 = Decrement(x=w515) -> (x-1=w520:u16)
              n264 = Scale By Power Of 2(n=w520, x=3) -> (x*2^n=w524:i32)
              n265 = Select(t=1, s=w521, f=w524) -> (s? t:f=w516:i32)
              n266 = local read "Title nID"() -> (w509:i32)
              n267 = Bundle By Name(cluster=w512, "det time"=w513, "FilterWidth"=w516, "reset cfs"=TRUE ("Bundle Element"), "n averaged"=0 ("Bundle Element"), "tf previous"=timestamp(0 s since 1904-01-01)) -> (w519:T16)
              n268 = Number To Decimal String(number=w509) -> (decimal integer string=w504:string)  [unwired: 1 in]
              n269 = Index Array(array=string[] ["1/1", "1/3", "1/6", "1/12", "1/24"], index=w515) -> (element=w517:string)
              n270 = call "CRYGet Window Title Message.vi"("No"=0 ("Error No"), "Kind"="RTA") -> ("Multibyte String"=w505:string)  [unwired: 4 in, 5 out]
              n271 = Concatenate Strings(w517, w505, "-" ("string"), w504) -> (w508:string)
              n272 = property class="VI"("Front Panel.Title"=w508) -> ()  [unwired: 2 in, 2 out]
            }
          }
        }
        frame 9 {
          n273 = Unbundle By Name(w537) -> ("Signal Path"=w536:i32)
          n274 = Not Equal?(x=w536, y=w532) -> (x != y?=w528:bool)
          n275 = Or(x=w525, y=w528) -> (x .or. y?=w527:bool)
          n276 = case shown="True" w527 {
            tunnel: w534 -> [w538 w546]
            tunnel: [w538 w545] -> w533
            tunnel: w532 -> [_ w544]
            tunnel: w531 -> [_ w543]
            tunnel: w530 -> [_ w542]
            tunnel: w526 -> [w539 w541]
            tunnel: [w539 w540] -> w529
            frame False {
            }
            frame True {
              n277 = stacked-sequence {
                tunnel: w546 -> [_ w610 _]
                tunnel: [_ w609 _] -> w545
                tunnel: w544 -> [_ w608 _]
                tunnel: w543 -> [_ w607 _]
                tunnel: w542 -> [_ w606 _]
                tunnel: w541 -> [_ w605 _]
                tunnel: [_ w604 _] -> w540
                frame #0 {
                  n278 = local read "Audio Driver"() -> (w547:u16)
                  n279 = case shown="2" w547 {
                    frame 2 {
                      n280 = local read "ASIO_Inited"() -> (w550:bool)
                      n281 = case shown="True" w550 {
                        frame False {
                        }
                        frame True {
                          n282 = local read "Channel In"() -> (w551:u16)
                          n283 = local read "Asio OCI"() -> (w552:u32)
                          n284 = local write "ASIO_Inited"(FALSE ("ASIO_Inited")) -> ()
                          n285 = call "CRYASIO Close Cur Channel & Dev.vi"("Limit"=w552, "isInput?"=TRUE, "Channel Out"=w551) -> ()  [unwired: 9 in]
                        }
                      }
                      n286 = local read "Rcv Idx"() -> (w549:u16)
                      n287 = local read "isMain"() -> (w548:bool)
                      n288 = call "CRYClear Main Receiver Array.vi"("isMain"=w548, "Rcv Idx"=w549) -> ()  [unwired: 10 in]
                    }
                    frame 0, Default {
                      w557 = 0.0 ("timeOut")
                      w558 = u8 0 ("nSampleFreq")
                      w559 = u32 0 ("nSampleFreq")
                      n289 = local read "Device In"() -> (w556:u16)
                      n290 = local read "taskID"() -> (w555:u32)
                      n291 = dll-call lib="D:/A_CRYSoundLab_Work/CRY6181/CRYSound.dll" fn="GVContinueRecord"("DeviceID"=w556, "nSampleFreq"=w559, "nChannels"=w559, "BitDepth"=w559, "TimeRate"=w557, "mode"=w559, "nBufferUse"=w559, "RealTime"=w559, "timeOut"=w557, "RecData"=i32[] [], "RecDataLen"=w559, "OverHead"=w558, "StartFlag"=w558, "PauseFlag"=w558, "ChangeFlag"=w558, "taskID"=w555) -> ()  [unwired: 10 in, 12 out]
                    }
                  }
                }
                frame #1 {
                  w563 = 4194303.0  # 2^22 - 1
                  n292 = local read "Calibration in"() -> (w580:string)
                  n293 = local read "Hardware in"() -> (w581:string)
                  n294 = property on="Signal Path" class="Ring (strict)"() -> ("RingText.Text"=w578:string)  [unwired: 2 in, 2 out]
                  n295 = case shown="False" w607 {
                    tunnel: [w618 "dB ref."] -> w585
                    tunnel: ["" ("prefix In") "prefix In"] -> w602
                    tunnel: [w616 "Y Units"] -> w584
                    tunnel: w606 -> [_ _]
                    tunnel: [w619 "Sens"] -> w601
                    tunnel: w578 -> [w617 _]
                    frame False {
                      n296 = call "CRYGet Current Calibration Info.vi"("Is Input?"=TRUE, "Signal Type Name"=w617) -> ("Calibration All Cluster"=w615:T12)  [unwired: 9 out]
                      n297 = Unbundle By Name(w615) -> ("Sens Curve"=w620:T6)
                      n298 = Unbundle By Name(w620) -> ("Curve"=w622:cluster{"x":dbl, "y":dbl, "z":dbl}[], "Y unit"=w616:string, "Y dB ref"=w618:dbl)
                      n299 = Index Array(array=w622) -> (element=w623:cluster{"x":dbl, "y":dbl, "z":dbl})  [unwired: 1 in]
                      n300 = Unbundle By Name(w623) -> ("y"=w619:dbl)
                      n301 = local write "dB ref."(w618) -> ()
                      n302 = local write "Sens"(w619) -> ()
                    }
                    frame True {
                    }
                  }
                  n303 = Search/Split String(string=w584, search string/char (-)="/" ("search char (-)")) -> (substring before match=w593:string, match + rest of string=w591:string, offset of match=w595:i32)  [unwired: 1 out]
                  n304 = String Subset(string=w591, offset (0)=1) -> (substring=w590:string)  [unwired: 1 in]
                  n305 = Greater Or Equal To 0?(x=w595) -> (x >= 0?=w594:bool)
                  n306 = call "CRYGet Hardware Info From Signal Type.vi"("Calibration In"=w580, "Hardware In"=w581, "Signal Type"=w578, "In/Out?"=TRUE) -> ("Channel Info Out"=w577:T15)  [unwired: 5 in, 2 out]
                  n307 = Unbundle By Name(w577) -> ("ID"=w597:i32, "Hardware Ch ID"=w565:u8, "Sampling Rate (Hz)"=w570:u32, "Bit Depth"=w569:u32, "Audio Driver"=w566:u16, "Device Name"=w567:string, "Vmax (V)"=w561:dbl)
                  n308 = Select(t=w590, s=w594, f=w593) -> (s? t:f=w583:string)
                  n309 = local write "Y Units"(w583) -> ()
                  n310 = local write "Device In"(w597) -> ()
                  n311 = local write "Sampling rate"(w570) -> ()
                  n312 = local write "Bits"(w569) -> ()
                  n313 = local write "Channel In"(w565) -> ()
                  n314 = Divide(x=w561, y=w601) -> (x/y=w600:dbl)
                  n315 = Divide(x=w600, y=w563) -> (x/y=w562:dbl)
                  n316 = call "CRYUnit Prefix to Multiplier.vi"("unit prefix"=w602) -> ("multiplier"=w603:dbl)  [unwired: 4 out]
                  n317 = To Double Precision Float(number=w570) -> (double precision float=w571:dbl)
                  n318 = To Long Integer(number=w569) -> (32bit integer=w572:i32)
                  n319 = Equal To 0?(x=w565) -> (x = 0?=w598:bool)
                  n320 = Multiply(x=w603, y=w585) -> (x*y=w599:dbl)
                  n321 = Bundle(w571, "32bit integer"=2, w572) -> (w574:cluster{dbl, "32bit integer":i32, i32})  [unwired: 1 in]
                  n322 = local write "Device Name"(w567) -> ()
                  n323 = local write "Audio Driver"(w566) -> ()
                  n324 = call "CRYGet Initialized WFM Array.vi"("Sound Format"=w574, "Time(s)"=0.05) -> ("initialized array"=w576:i32[])  [unwired: 8 in, 5 out]
                  n325 = Format Into String(format string="dB re %.p %s", w585, w583) -> (resulting string=w589:string)  [unwired: 2 in, 1 out]
                  n326 = Concatenate Strings("Amplitude [" ("string"), w589, "]" ("string")) -> (w582:string)
                  n327 = case shown="0, Default" w566 {
                    tunnel: w565 -> [_ w613]
                    frame 0, Default {
                      n328 = local read "Rcv Idx"() -> (w611:u16)
                      n329 = call "CRYUpdate Receiver Index.vi"("Chn Idx"=-1, "Receiver_Index"=w611) -> ()  [unwired: 9 in]
                    }
                    frame 2 {
                      n330 = local read "Rcv Idx"() -> (w614:u16)
                      n331 = call "CRYUpdate Receiver Index.vi"("Chn Idx"=w613, "Receiver_Index"=w614) -> ()  [unwired: 9 in]
                    }
                  }
                  n332 = Bundle By Name(cluster=w605, "Signal Path"=w608) -> (w604:T20)
                  n333 = local write "initialized array"(w576) -> ()
                  n334 = Bundle By Name(cluster=w610, "reset cfs"=TRUE, "ch left"=w598, "cal factor"=w562, "db-pr factor"=w599, "max level"=w561, "tf previous"=timestamp(0 s since 1904-01-01)) -> (w609:T16)
                  n335 = property on="Spectrum" class="XYGraph (strict)"("YScale.NameLbl.Text"=w582) -> ()  [unwired: 2 in, 2 out]
                }
                frame #2 {
                  n336 = local read "Audio Driver"() -> (w630:u16)
                  n337 = local read "ASIO_Inited"() -> (w631:bool)
                  n338 = case shown="2" w630 {
                    tunnel: w631 -> [w634 _]
                    frame 2 {
                      n339 = case shown="False" w634 {
                        frame False {
                          n340 = local read "Device Name"() -> (w641:string)
                          n341 = local read "Sampling rate"() -> (w639:dbl)
                          n342 = local read "Channel In"() -> (w640:u16)
                          n343 = local read "Bits"() -> (w638:i32)
                          n344 = local write "Buf Cnt"(-1 ("Buf Cnt")) -> ()
                          n345 = call "CRYASIO In & Init & Start.vi"("Bit Depth"=w638, "Sampling Rate"=w639, "Channel Index"=w640, "Device Name"=w641) -> ("bResult"=w636:bool, "ASIO Opend Channel Index"=w637:u32)  [unwired: 6 in]
                          n346 = local write "ASIO_Inited"(w636) -> ()
                          n347 = local write "Asio OCI"(w637) -> ()
                        }
                        frame True {
                        }
                      }
                      n348 = local read "Rcv Idx"() -> (w633:u16)
                      n349 = call "CRYSet Main Receiver Array.vi"("Rcv Idx"=w633) -> ("Is Main?"=w632:bool)  [unwired: 10 in]
                      n350 = local write "isMain"(w632) -> ()
                    }
                    frame 0, Default {
                      n351 = local write "start_flg"(u8 1 ("start_flg")) -> ()
                    }
                  }
                  n352 = local write "Remain Data"(i32[] [] ("Remain Data")) -> ()
                }
              }
            }
          }
        }
        frame 10 {
          n353 = Unbundle By Name(w654) -> ("Weighting"=w653:i32)
          n354 = Not Equal?(x=w653, y=w649) -> (x != y?=w647:bool)
          n355 = Compound Arithmetic op=OR(w648, w647) -> (w645:bool)
          n356 = case shown="True" w645 {
            tunnel: w651 -> [w656 w663]
            tunnel: [w656 w662] -> w650
            tunnel: w649 -> [_ w661]
            tunnel: w646 -> [_ w660]
            tunnel: w644 -> [w655 w657]
            tunnel: [w655 w657] -> w643
            frame False {
            }
            frame True {
              n357 = case shown="True" "分支常量\n（见即时帮助）" {
                tunnel: w661 -> [w664 _]
                tunnel: [w665 w667] -> _
                tunnel: w660 -> [_ w669]
                frame False {
                  # "dB"
                  n358 = Increment(x=w664) -> ()  [unwired: 1 out]
                  n359 = Index Array(array="Freq, A, B, C wgt.", index (row)=w664) -> (element=w665:dbl[])  [unwired: 1 in]
                }
                frame True {
                  # "linear"
                  n360 = Index Array(array="A-weights table", index (row)=w669) -> (element=w667:dbl[])  [unwired: 1 in]
                }
              }
              n361 = Bundle By Name(cluster=w663, "new weight"=TRUE) -> (w662:T16)
            }
          }
        }
        frame 11 {
          n362 = Unbundle By Name(w681) -> ("Time Weighting"=w680:i32)
          n363 = Not Equal?(x=w680, y=w675) -> (x != y?=w678:bool)
          n364 = Or(x=w679, y=w678) -> (x .or. y?=w673:bool)
          n365 = case shown="True" w673 {
            tunnel: w677 -> [w683 w690]
            tunnel: [w683 w689] -> w676
            tunnel: w675 -> [_ w691]
            tunnel: w674 -> [_ w692]
            tunnel: w671 -> [w682 w684]
            tunnel: [w682 w684] -> w670
            frame False {
            }
            frame True {
              n366 = case shown="2" w691 {
                tunnel: [0.125 ("DetectorTime") 1.0 ("DetectorTime") w700] -> w687
                tunnel: [u8 2 ("Write Attribute") u8 2 ("Write Attribute") u8 0 ("Write Attribute")] -> w685
                tunnel: w692 -> [_ _ w700]
                tunnel: [u8 0 ("Numeric Text.Format & Precision:Precision") u8 1 ("Numeric Text.Format & Precision:Precision") u8 1 ("Numeric Text.Format & Precision:Precision")] -> w686
                frame 0, Default {
                }
                frame 1 {
                }
                frame 2 {
                }
              }
              n367 = property on="Avg. Time(sec)" class="DigNum (strict)"("NumText.Precision"=w686) -> ()  [unwired: 2 in, 2 out]
              n368 = Tick Count (ms)() -> (millisecond timer value=w688:u32)
              n369 = property on="Avg. Time(sec)" class="DigNum (strict)"("Disabled"=w685) -> ()  [unwired: 2 in, 2 out]
              n370 = Bundle By Name(cluster=w690, "det time"=w687, "ref time"=w688) -> (w689:T16)
              n371 = local write "Avg. Time(sec)"(w687) -> ()
            }
          }
        }
        frame 12 {
          n372 = Unbundle By Name(w710) -> ("Avg. Time(sec)"=w709:dbl)
          n373 = Not Equal?(x=w709, y=w706) -> (x != y?=w705:bool)
          n374 = case shown="True" w705 {
            tunnel: w708 -> [w712 w719]
            tunnel: [w712 w713] -> w702
            tunnel: w707 -> [_ w718]
            tunnel: w706 -> [_ w717]
            tunnel: w704 -> [w711 w716]
            tunnel: [w711 w716] -> w703
            frame False {
            }
            frame True {
              n375 = case shown="2" w718 {
                tunnel: w719 -> [w720 w724]
                tunnel: [w720 w723] -> w714
                tunnel: w717 -> [_ w722]
                frame Default {
                }
                frame 2 {
                  n376 = Tick Count (ms)() -> (millisecond timer value=w721:u32)
                  n377 = Bundle By Name(cluster=w724, "det time"=w722, "ref time"=w721) -> (w723:T16)
                }
              }
              n378 = Bundle By Name(cluster=w714, "reset cfs"=TRUE) -> (w713:T16)
            }
          }
        }
        frame Default {
          n379 = Unbundle By Name(w736) -> ("acquire"=w725:bool, "n averaged"=w731:i32)
          n380 = Multiply(x=w731, y=0.05) -> (x*y=w732:dbl)
          n381 = Less?(x=w726, y=w732) -> (x < y?=w728:bool)
          n382 = Equal To 0?(x=w737) -> (x = 0?=w733:bool)
          n383 = And(x=w733, y=w728) -> (x .and. y?=w729:bool)
          n384 = case shown="True" w729 {
            tunnel: w736 -> [w748 w763]
            tunnel: [w748 w762] -> w727
            tunnel: w735 -> [_ w760]
            tunnel: w726 -> [w747 w758]
            tunnel: w725 -> [w746 _]
            frame False {
              n385 = case shown="True" w746 {
                tunnel: w748 -> [_ w754]
                tunnel: w747 -> [_ w751]
                frame False {
                }
                frame True {
                  n386 = Unbundle By Name(w754) -> ("ref time"=w753:u32)
                  n387 = Tick Count (ms)() -> (millisecond timer value=w755:u32)
                  n388 = Subtract(x=w755, y=w753) -> (x-y=w756:u32)
                  n389 = Multiply(x=w756, y=0.001) -> (x*y=w750:dbl)
                  n390 = Less?(x=w751, y=w750) -> (x < y?=w752:bool)
                  n391 = Select(t=w751, s=w752, f=w750) -> (s? t:f=w749:dbl)
                  n392 = local write "Elapsed Time"(w749) -> ()
                }
              }
            }
            frame True {
              w761 = FALSE ("acquire")
              n393 = case shown="False" w760 {
                frame False {
                  n394 = local write "OK"(TRUE ("OK")) -> ()
                }
                frame True {
                }
              }
              n395 = local write "Elapsed Time"(w758) -> ()
              n396 = Bundle By Name(cluster=w763, "acquire"=w761, "n averaged"=0) -> (w762:T16)
              n397 = local write "Start"(w761) -> ()
              n398 = local write "Continue"(w761) -> ()
            }
          }
          n399 = disable-structure shown="Disabled" {
            frame Disabled {
              n400 = Wait (ms)(milliseconds to wait=u32 10) -> ()  [unwired: 1 out]
            }
            frame Enabled {
            }
          }
          n401 = case shown="True" w728 {
            tunnel: w727 -> [w741 w745]
            tunnel: [w741 w743] -> w734
            frame False {
            }
            frame True {
              n402 = Bundle By Name(cluster=w745, "reset cfs"=TRUE, "n averaged"=0) -> (w743:T16)
            }
          }
        }
      }
      n403 = Not(x=w270) -> (.not. x?=w269:bool)
    }
    n404 = Unbundle By Name(w224) -> ("reset cfs"=w231:bool, "acquire"=w190:bool)
    n405 = case shown="True" w190 {
      tunnel: w224 -> [w769 w840]
      tunnel: [w769 w798] -> w232
      tunnel: [w771 w869] -> w238
      tunnel: w237 -> [w771 w841]
      tunnel: w235 -> [w773 w868]
      tunnel: [w773 w867] -> w234
      tunnel: [w772 w846] -> w233
      tunnel: w191 -> [w772 w845]
      tunnel: w231 -> [_ w853]
      tunnel: w190 -> [_ w864]
      tunnel: w223 -> [w770 w859]
      tunnel: [w770 w858] -> w222
      tunnel: w189 -> [w768 _]
      frame False {
        n406 = Unbundle By Name(w768) -> ("acquire"=w767:bool)
        n407 = case shown="True" w767 {
          frame False {
          }
          frame True {
            w787 = 0.0 ("timeOut")
            w786 = u8 0 ("nSampleFreq")
            w785 = u32 0 ("nSampleFreq")
            n408 = local read "Device In"() -> (w788:u16)
            n409 = local read "taskID"() -> (w789:u32)
            n410 = dll-call lib="D:/A_CRYSoundLab_Work/CRY6181/CRYSound.dll" fn="GVContinueRecord"("DeviceID"=w788, "nSampleFreq"=w785, "nChannels"=w785, "BitDepth"=w785, "TimeRate"=w787, "mode"=w785, "nBufferUse"=w785, "RealTime"=w785, "timeOut"=w787, "RecData"=i32[] [], "RecDataLen"=w785, "OverHead"=w786, "StartFlag"=w786, "PauseFlag"=w786, "ChangeFlag"=w786, "taskID"=w789) -> ()  [unwired: 10 in, 12 out]
          }
        }
        n411 = local read "Audio Driver"() -> (w766:u16)
        n412 = case shown="2" w766 {
          frame 2 {
            n413 = local read "Rcv Idx"() -> (w775:u16)
            n414 = local read "ASIO_Inited"() -> (w777:bool)
            n415 = call "CRYCheck Main Receiver.vi"("Rcv Idx"=w775) -> ("Is Main?"=w776:bool)  [unwired: 10 in]
            n416 = And(x=w777, y=w776) -> (x .and. y?=w774:bool)
            n417 = case shown="False" w774 {
              tunnel: w775 -> [_ w780]
              frame False {
                n418 = local write "Buf Cnt"(-1 ("Buf Cnt")) -> ()
              }
              frame True {
                n419 = local read "Asio OCI"() -> (w783:u32)
                n420 = call "CRYASIO Receive Data.vi"("Rcv Idx"=w780, "Limit"=w783, "Data Length"=2048, "Last Remain Buffer"=i32[] []) -> ()  [unwired: 5 in, 3 out]
              }
            }
            n421 = local write "isMain"(w776) -> ()
            n422 = Wait (ms)(milliseconds to wait=u32 10) -> ()  [unwired: 1 out]
          }
          frame 0, Default {
          }
        }
      }
      frame True {
        w803 = T2 0 items=["custom..."=0, "V"=1, "A"=21, "Pa"=2, "N"=20, "g"=3, "m/s^2"=4, "m/s"=5, "m"=6, "mm/s"=12, "mm"=13, "micron/s"=14, "micron"=15, "in/s^2"=7, "in/s"=8, "in"=9, "mil/s"=10, "mil"=11, "rad/s^2"=16, "rad/s"=17, "rad"=18, "deg/s^2"=26, "deg/s"=27, "deg"=28, "RPM"=22, "cycle/s^2"=23, "Hz"=24, "cycle"=25, "strain"=19] ("engineering units")
        w820 = 1  # ???
        w847 = FALSE
        # "????????"
        n423 = Unbundle By Name(w840) -> ("n averaged"=w843:i32, "reset cfs"=w804:bool, "reset throw"=w861:bool, "halt acq"=w857:bool, "cal factor"=w792:dbl, "avg type"=w805:i32, "ref time"=w856:u32, "new weight"=w854:bool)  [unwired: 3 out]
        "cal factor" <- w792
        n424 = local read "Audio Driver"() -> (w807:u16)
        n425 = Greater Than 0?(x=w805) -> (x > 0?=w844:bool)
        n426 = local read "Avg. Time(sec)"() -> (w838:dbl)
        n427 = local read "Sampling rate"() -> (w837:dbl)
        n428 = local read "initialized array"() -> (w834:i32[])
        n429 = Equal To 0?(x=w807) -> (x = 0?=w816:bool)
        n430 = local read "Sampling rate"() -> (w831:dbl)
        n431 = Select(t=0.1 ("x"), s=w816, f=0.05 ("x")) -> (s? t:f=w813:dbl)
        n432 = local read "Channel In"() -> (w806:u16)
        n433 = local read "Device In"() -> (w830:u16)
        n434 = local read "Bits"() -> (w833:i32)
        n435 = Multiply(x=w813, y=w837) -> (x*y=w836:dbl)
        n436 = Multiply(x=w838, y=w837) -> (x*y=w835:dbl)
        n437 = Boolean To (0,1)(Boolean=w804) -> (0, 1=w817:i16)
        n438 = To Long Integer(number=w836) -> (32bit integer=w839:i32)
        n439 = To Long Integer(number=w835) -> ()  [unwired: 1 out]
        n440 = To Unsigned Long Integer(number=w831) -> (unsigned 32bit integer=w832:u32)
        n441 = Increment(x=w843) -> (x+1=w842:i32)
        n442 = while {
          tunnel: w833 -> [w891]
          tunnel: w832 -> [w892]
          tunnel: w830 -> [w893]
          tunnel: w820 -> [w875]
          tunnel: w857 -> [w886]
          shift-left: 0 -> [w895]
          shift-right: [w873] -> _
          tunnel: u8 0 ("OverHead") -> [w887]
          shift-left: i32[] [] -> [w897]
          shift-right: [w896] -> w824
          tunnel: w834 -> [w890]
          tunnel: 0.05 ("TimeRate") -> [w889]
          tunnel: 0.0 ("timeOut") -> [w888]
          shift-right: [w884] -> _
          shift-left: u8 0 ("OverHead") -> [w885]
          shift-right: [w882] -> _
          shift-left: w817 -> [w883]
          tunnel: w839 -> [w881]
          tunnel: [w880] -> w808
          tunnel: [w877] -> w851
          tunnel: w807 -> [w876]
          tunnel: w806 -> [w870]
          stop <- w894 continue-if-true
          n443 = case shown="0, Default" w876 {
            tunnel: w897 -> [_ w967]
            tunnel: [w907 w966] -> w896
            tunnel: w895 -> [w910 w965]
            tunnel: [w909 w938] -> w873
            tunnel: w875 -> [_ _]
            tunnel: w893 -> [_ w964]
            tunnel: w892 -> [_ w963]
            tunnel: w891 -> [_ w962]
            tunnel: w890 -> [_ w961]
            tunnel: w889 -> [_ w960]
            tunnel: w888 -> [_ w959]
            tunnel: w887 -> [_ w958]
            tunnel: w885 -> [w903 w948]
            tunnel: [w902 w947] -> w884
            tunnel: w883 -> [_ w946]
            tunnel: [i16 0 i16 0] -> w882
            tunnel: w881 -> [w911 w944]
            tunnel: [FALSE w941] -> w880
            tunnel: [u32 0 ("nBufferUse") w940] -> w877
            tunnel: w870 -> [w900 _]
            frame 2 {
              n444 = local read "ASIO_Inited"() -> (w908:bool)
              n445 = local read "Rcv Idx"() -> (w899:u16)
              n446 = call "CRYCheck Main Receiver.vi"("Rcv Idx"=w899) -> ("Is Main?"=w898:bool)  [unwired: 10 in]
              n447 = case shown="True" w908 {
                tunnel: w911 -> [w912 w920]
                tunnel: [0 ("Over Load") w919] -> w904
                tunnel: [w914 w918] -> w907
                tunnel: w900 -> [_ w917]
                tunnel: w898 -> [_ w916]
                frame False {
                  n448 = Initialize Array(0 ("element"), w912) -> (w914:i32[])
                }
                frame True {
                  n449 = case shown="False" w916 {
                    tunnel: w920 -> [w926 w934]
                    tunnel: [w925 w933] -> w919
                    tunnel: [w923 w932] -> w918
                    tunnel: w917 -> [_ w930]
                    frame True {
                      n450 = local read "Remain Data"() -> (w927:i32[])
                      n451 = local read "Asio OCI"() -> (w924:u32)
                      n452 = local read "Rcv Idx"() -> (w921:u16)
                      n453 = call "CRYASIO Receive Data.vi"("Rcv Idx"=w921, "Limit"=w924, "Data Length"=w926, "Last Remain Buffer"=w927) -> ("Over Load"=w925:i32, "Data Out"=w923:i32[], "Remain Data"=w922:i32[])  [unwired: 5 in]
                      n454 = local write "Remain Data"(w922) -> ()
                    }
                    frame False {
                      n455 = local read "Remain Data"() -> (w935:i32[])
                      n456 = local read "Buf Cnt"() -> (w928:i32)
                      n457 = call "CRYASIO Receive Global Data.vi"("buf count"=w928, "Chn Idx"=w930, "Data Length"=w934, "Last Remain Buffer"=w935) -> ("Over Load"=w933:i32, "bufCount"=w929:i32, "Data Out"=w932:i32[], "Remain Data"=w931:i32[])  [unwired: 4 in]
                      n458 = local write "Remain Data"(w931) -> ()
                      n459 = local write "Buf Cnt"(w929) -> ()
                    }
                  }
                }
              }
              n460 = local write "isMain"(w898) -> ()
              n461 = Increment(x=w910) -> (x+1=w909:i32)
              n462 = Add(x=w904, y=w903) -> (x+y=w902:i32)
            }
            frame 0, Default {
              w939 = u32 0 ("RecDataLen")
              (unwired) u8 1 ("StartFlag")
              n463 = local read "start_flg"() -> (w936:u8)
              n464 = dll-call lib="D:/A_CRYSoundLab_Work/CRY6181/CRYSound.dll" fn="GVContinueRecord"("DeviceID"=w964, "nSampleFreq"=w963, "nChannels"=u32 2, "BitDepth"=w962, "TimeRate"=w960, "mode"=u32 0, "timeOut"=w959, "RecData"=w961, "RecDataLen"=w939, "OverHead"=w939, "StartFlag"=w936, "PauseFlag"=w958, "ChangeFlag"=w946, "taskID"="taskID") -> ("return type"=w937:u32, "nBufferUse"=w940:u32, "RealTime"=w954:u32, "RecData"=w956:i32[], "RecDataLen"=w953:u32, "OverHead"=w949:u8, "taskID"=w951:u32)  [unwired: 11 in, 6 out]
              n465 = To Unsigned Byte Integer(number=w940) -> (unsigned 8bit integer=→"Buffer":u8)
              n466 = To Unsigned Byte Integer(number=w954) -> (unsigned 8bit integer=→"Real Time":u8)
              n467 = local write "taskID"(w951) -> ()
              n468 = Not Equal To 0?(x=w937) -> (x != 0?=w941:bool)
              n469 = Equal To 0?(x=w953) -> (x = 0?=w957:bool)
              n470 = Add(x=w949, y=w948) -> (x+y=w947:i32)
              n471 = case shown="False" w957 {
                tunnel: w956 -> [w972 _]
                tunnel: w967 -> [w976 w979]
                tunnel: [w975 w979] -> w966
                tunnel: w965 -> [w974 w978]
                tunnel: [w973 w978] -> w938
                tunnel: w944 -> [w970 _]
                frame False {
                  n472 = Array Subset(array=w972, length=w970) -> (w971:i32[])  [unwired: 1 in]
                  n473 = Increment(x=w974) -> (x+1=w973:i32)
                  n474 = Build Array (concatenate)(w976, w971) -> (w975:i32[])
                }
                frame True {
                  n475 = Wait (ms)(milliseconds to wait=u32 21) -> ()  [unwired: 1 out]
                }
              }
              n476 = case shown="2" w937 {
                frame 0, Default {
                }
                frame 2 {
                  w968 = FALSE ("Start")
                  n477 = local write "start_flg"(u8 0 ("start_flg")) -> ()
                  n478 = local write "Continue"(w968) -> ()
                  n479 = local write "Start"(w968) -> ()
                }
              }
            }
          }
          n480 = local read "OK"() -> (w878:bool)
          n481 = local read "start_flg"() -> (w872:u8)
          n482 = Less?(x=w873, y=w875) -> (x < y?=w874:bool)
          n483 = local read "Cancel"() -> (w879:bool)
          n484 = Equal To 0?(x=w872) -> (x = 0?=w871:bool)
          n485 = Compound Arithmetic op=AND(invert w886, w874, invert w879, invert w878, invert w871) -> (w894:bool)
        }
        n486 = Bundle By Name(cluster=w840, "n averaged"=w842) -> (w800:T16)
        n487 = local read "Channel In"() -> (w825:u16)
        n488 = Equal To 0?(x=w807) -> (x = 0?=w812:bool)
        n489 = Select(t=2 ("N channels"), s=w812, f=1 ("N channels")) -> (s? t:f=w809:i32)
        n490 = call "CRYChannel separate buffer array.vi"("N channels"=w809, "Buffer array in"=w824) -> ("First right channel"=w822:i32[], "First left channel"=w821:i32[])  [unwired: 8 out]
        n491 = Equal To 0?(x=w825) -> (x = 0?=w823:bool)
        n492 = Select(t=w821, s=w823, f=w822) -> (s? t:f=w794:i32[])
        n493 = Multiply(x=w794, y=w792) -> (x*y=w793:dbl[])
        n494 = Select(t=0 ("Iteration"), s=w861, f=1 ("Iteration")) -> (s? t:f=w850:i32)
        n495 = call "CRYData throw-away decide.vi"("Iteration"=w850, "Buffer use (%)"=w851) -> ("Portion of data processed (%)"=w849:dbl, "Suppress processing"=w848:bool)  [unwired: 1 in, 7 out]
        n496 = Multiply(x=5.0, y=w849) -> ()  [unwired: 1 out]
        n497 = Compound Arithmetic op=OR(w808, w853, w854) -> (w852:bool)
        n498 = Compound Arithmetic op=OR(w848, w808, w857) -> (w862:bool)
        n499 = Not Or(1:w844, 2:w853) -> (0:w855:bool)
        n500 = case shown="True" w855 {
          tunnel: w856 -> [_ w980]
          frame False {
          }
          frame True {
            n501 = disable-structure shown="Disabled" {
              disable-tunnel: w980 -> [w984 _]
              frame Disabled {
                n502 = Tick Count (ms)() -> (millisecond timer value=w985:u32)
                n503 = Subtract(x=w985, y=w984) -> (x-y=w983:u32)
                n504 = Multiply(x=w983, y=0.001) -> (x*y=→"Elapsed Time":dbl)
              }
              frame Enabled {
              }
            }
          }
        }
        n505 = Compound Arithmetic op=AND(invert w808, invert w857, w864) -> (w863:bool)
        n506 = Bundle By Name(cluster=w800, "reset cfs"=w847, "halt acq"=w847, "reset throw"=w847, "acquire"=w863) -> (w799:T16)
        n507 = local read "Weighting"() -> (w795:i32)
        n508 = local read "dB ref."() -> (w791:dbl)
        n509 = Bundle By Name(cluster="channel info", "sensor sensitivity [mV/EU]"=1000.0, "engineering units"=w803, "dB reference [EU]"=w791, "custom label"="EU", "weighting filter"=w795, "pregain [dB]"=0.0) -> (w796:T1)
        n510 = case shown="False" w862 {
          tunnel: w793 -> [w989 _]
          tunnel: [w999 w1070] -> w869
          tunnel: w841 -> [_ w1070]
          tunnel: w868 -> [w1026 w1069]
          tunnel: [w1025 w1069] -> w867
          tunnel: w852 -> [w1023 _]
          tunnel: w859 -> [w1022 w1068]
          tunnel: [w1021 w1068] -> w858
          tunnel: [w1019 w1067] -> w846
          tunnel: w845 -> [_ w1067]
          tunnel: w807 -> [w1009 _]
          tunnel: w805 -> [w1008 _]
          tunnel: w804 -> [_ _]
          tunnel: w796 -> [w1006 _]
          tunnel: w799 -> [w1004 w1066]
          tunnel: [w1003 w1066] -> w798
          frame False {
            n511 = local read "Sampling rate"() -> (w998:dbl)
            n512 = Unbundle By Name(w1004) -> ("tf previous"=w1005:timestamp)
            n513 = case shown="2" w1009 {
              tunnel: w989 -> [w1029 w1031]
              tunnel: [w1029 w1030] -> w990
              frame 0, Default {
              }
              frame 2 {
                n514 = Divide(x=w1031, y=512.0 ("low frequency")) -> (x/y=w1030:dbl[])
              }
            }
            n515 = Not(x=w1023) -> (.not. x?=w1024:bool)
            n516 = local read "Time Weighting"() -> (w1012:i32)
            n517 = Array Size(array=w990) -> (size(s)=w1002:i32)
            n518 = Decrement(x=w1002) -> (x-1=w997:i32)
            n519 = Reciprocal(x=w998) -> (1/x=w995:dbl)
            n520 = Add(x=w1005, y=w995) -> (x+y=w1000:timestamp)
            n521 = Multiply(x=w995, y=w997) -> (x*y=w996:dbl)
            n522 = Bundle By Name("Y"=w990, "dt"=w995, "t0"=w1000) -> (w1018:waveform(dbl))  [unwired: 1 in]
            n523 = Bundle By Name(cluster=T18 {"low frequency"=20.0, "high frequency"=8000.0} ("frequency range [Hz]"), "low frequency"=8.0, "high frequency"=w998) -> (w994:T18)
            n524 = Add(x=w1000, y=w996) -> (x+y=w1001:timestamp)
            n525 = case shown="2" w1012 {
              tunnel: [enum16{"Slow", "Fast", "Impulse", "Custom"}."Fast" ("mode") enum16{"Slow", "Fast", "Impulse", "Custom"}."Slow" ("mode") enum16{"Slow", "Fast", "Impulse", "Custom"}."Custom" ("mode")] -> w1014
              frame 0, Default {
              }
              frame 1 {
              }
              frame 2 {
              }
            }
            n526 = case shown="0, Default" w1008 {
              tunnel: [T19."Linear" ("averaging type") T19."Exponential" ("averaging type")] -> w1007
              frame 0, Default {
              }
              frame 1 {
              }
            }
            n527 = local read "Avg. Time(sec)"() -> (w1015:dbl)
            n528 = Bundle By Name(cluster=w1004, "tf previous"=w1001) -> (w1003:T16)
            n529 = property on="Weighting" class="Ring (strict)"() -> ("Value"=w986:i32)  [unwired: 2 in, 2 out]
            n530 = case shown="1, Default" w986 {
              selector: w986 -> [_ w1034]
              tunnel: [w1033 w1035] -> w988
              tunnel: w1018 -> [w1033 w1036]
              frame 0 {
              }
              frame 1, Default {
                n531 = Set Waveform Attribute(5:w1034, 6:"NI_SV_WeightingFilter" ("name"), 7:w1036) -> (3:w1035:waveform(dbl))  [unwired: 1 in, 2 out]
              }
            }
            n532 = Bundle By Name(cluster=T17 {" mode"=enum."Slow", "time constant [ms]"=125.0} ("exp avg settings"), "mode"=w1014, "time constant [ms]"=w1015) -> (w993:T17)
            n533 = local read "Octave Band"() -> (w992:u16)
            n534 = call-poly <vilib>:"SVL Scale Voltage to EU.vi"("channel info"=w1006, "signal [V]"=w988) -> ("scaled signal [EU]"=w987:waveform(dbl))  [unwired: 7 in, 2 out]
            n535 = call-poly <vilib>:"SVT Fractional-octave Analysis.vi"("scaled signal [EU]"=w987, "frequency range [Hz]"=w994, "bandwidth"=w992, "error in (no error)"=errorcluster {"status"=FALSE, "code"=0, "source"=""}, "averaging type"=w1007, "exp avg settings"=w993, "equal confidence level [dB]"="equal confidence level [dB]") -> ("octave spectrum"=w999:T7, "error out"=→"error out 2":errorcluster)  [unwired: 3 in, 4 out]
            n536 = Unbundle(w999) -> ("nominal frequencies [Hz]"=w1019:dbl[], "band power"=w1020:dbl[])
            n537 = case shown="True" w1024 {
              tunnel: w1026 -> [_ w1058]
              tunnel: w1020 -> [w1054 w1057]
              tunnel: [w1054 w1056] -> w1025
              frame False {
              }
              frame True {
                n538 = local read "A/M/M"() -> (w1055:i32)
                n539 = case shown="2" w1055 {
                  tunnel: w1058 -> [_ w1062 w1065]
                  tunnel: w1057 -> [w1059 w1061 w1064]
                  tunnel: [w1059 w1060 w1063] -> w1056
                  frame 0, Default {
                  }
                  frame 1 {
                    n540 = Max & Min(x=w1062, y=w1061) -> (max(x,y)=w1060:dbl[])  [unwired: 1 out]
                  }
                  frame 2 {
                    n541 = Max & Min(x=w1065, y=w1064) -> (min(x,y)=w1063:dbl[])  [unwired: 1 out]
                  }
                }
              }
            }
            n542 = case shown="False" w1023 {
              tunnel: w999 -> [w1044 _]
              tunnel: w1022 -> [w1042 w1053]
              tunnel: [w1043 w1053] -> w1021
              frame False {
                n543 = stacked-sequence {
                  tunnel: w1044 -> [w1045 _]
                  tunnel: [w1045 _] -> w1041
                  frame #0 {
                    "Spectrum" <- w1045
                  }
                  frame #1 {
                    n544 = control-ref of="Spectrum"() -> (w1047:refnum<vi>)
                    n545 = call "CRYPaint WaterMark.vi"("Type"="Small", "Graph Ref"=w1047) -> ()  [unwired: 10 in]
                  }
                }
                n546 = Increment(x=w1042) -> (x+1=w1043:i32)
                n547 = case shown="2" w1042 {
                  tunnel: w1041 -> [_ _]
                  frame 2 {
                    n548 = stacked-sequence {
                      frame #0 {
                        n549 = disable-structure shown="禁用" {
                          frame Disabled {
                            n550 = property on="Spectrum" class="XYGraph (strict)"("YScale.ScaleFit"=u8 0 ("Write Attribute")) -> ()  [unwired: 2 in, 2 out]
                          }
                          frame Enabled {
                          }
                        }
                      }
                      frame #1 {
                        n551 = Wait (ms)(milliseconds to wait=u32 5) -> ()  [unwired: 1 out]
                      }
                      frame #2 {
                        n552 = disable-structure shown="禁用" {
                          frame Disabled {
                            n553 = property on="Spectrum" class="XYGraph (strict)"() -> ("YScale.Maximum"=w1051:dbl)  [unwired: 2 in, 2 out]
                            n554 = Add(x=w1051, y=10.0) -> (x+y=w1050:dbl)
                            n555 = property on="Spectrum" class="XYGraph (strict)"("YScale.Maximum"=w1050) -> ()  [unwired: 2 in, 2 out]
                          }
                          frame Enabled {
                          }
                        }
                      }
                    }
                  }
                  frame Default {
                  }
                }
              }
              frame True {
              }
            }
          }
          frame True {
          }
        }
      }
    }
    n556 = property on="Spectrum" class="XYGraph (strict)"() -> ("CrsrList"=w196:T21)  [unwired: 2 in, 2 out]
    n557 = Index Array(array=w196, index #1=1 ("index"), index #2=0 ("index")) -> (element #1=w202:T22, element #2=w199:T22)
    n558 = Unbundle By Name(w202) -> ("Position.Y"=w195:dbl, "Position.X"=w197:dbl)
    n559 = Unbundle By Name(w199) -> ("Position.X"=w198:dbl, "Position.Y"=w194:dbl)
    n560 = Subtract(x=w197, y=w198) -> (x-y=w193:dbl)
    n561 = local write "delta_X"(w193) -> ()
    n562 = Subtract(x=w195, y=w194) -> (x-y=w192:dbl)
    n563 = local write "delta_Y"(w192) -> ()
    n564 = stacked-sequence {
      tunnel: ["cont loop"] -> w239
      tunnel: w232 -> [_]
      frame #0 {
      }
    }
  }
  "band power" <- w5
  "df Array" <- w4
  n565 = stacked-sequence {
    tunnel: w9 -> [_ _ _ _ _]
    frame #0 {
      w1077 = 0.0 ("timeOut")
      w1076 = u8 0 ("nSampleFreq")
      w1075 = u32 0 ("nSampleFreq")
      n566 = local read "Audio Driver"() -> (w1073:u16)
      n567 = local read "Device In"() -> (w1078:u16)
      n568 = local read "taskID"() -> (w1079:u32)
      n569 = case shown="2" w1073 {
        frame 2 {
          n570 = local read "ASIO_Inited"() -> (w1080:bool)
          n571 = case shown="True" w1080 {
            frame False {
            }
            frame True {
              n572 = local read "Channel In"() -> (w1081:u16)
              n573 = local read "Asio OCI"() -> (w1082:u32)
              n574 = local write "ASIO_Inited"(FALSE ("ASIO_Inited")) -> ()
              n575 = call "CRYASIO Close Cur Channel & Dev.vi"("Limit"=w1082, "isInput?"=TRUE, "Channel Out"=w1081) -> ()  [unwired: 9 in]
            }
          }
        }
        frame 0, Default {
        }
      }
      n576 = dll-call lib="D:/A_CRYSoundLab_Work/CRY6181/CRYSound.dll" fn="GVContinueRecord"("DeviceID"=w1078, "nSampleFreq"=w1075, "nChannels"=w1075, "BitDepth"=w1075, "TimeRate"=w1077, "mode"=w1075, "nBufferUse"=w1075, "RealTime"=w1075, "timeOut"=w1077, "RecData"=i32[] [], "RecDataLen"=w1075, "OverHead"=w1076, "StartFlag"=w1076, "PauseFlag"=w1076, "ChangeFlag"=w1076, "taskID"=w1079) -> ()  [unwired: 10 in, 12 out]
      n577 = local read "Rcv Idx"() -> (w1072:u16)
      n578 = local read "isMain"() -> (w1071:bool)
      n579 = call "CRYClear Main Receiver Array.vi"("isMain"=w1071, "Rcv Idx"=w1072) -> ()  [unwired: 10 in]
    }
    frame #1 {
      n580 = local read "Time Weighting"() -> (w1099:i32)
      n581 = local read "Octave Band"() -> (w1100:u16)
      n582 = local read "Avg. Time(sec)"() -> (w1098:dbl)
      n583 = local read "Weighting"() -> (w1096:i32)
      n584 = local read "Lin/Exp"() -> (w1097:i32)
      n585 = local read "Channel In"() -> (w1095:u16)
      n586 = property on="Signal Path" class="Ring (strict)"() -> ("RingText.Text"=w1094:string)  [unwired: 2 in, 2 out]
      n587 = global read "CRYMisc vis settings global.vi" "Rcv Index Array"() -> (w1087:T23)
      n588 = local read "Rcv Idx"() -> (w1085:u16)
      n589 = global read "CRYMisc vis settings global.vi" "RTA settings"() -> (w1090:T11)
      n590 = Bundle By Name(cluster=w1090, "octave"=w1100, "det time"=w1099, "det sec"=w1098, "lin/exp"=w1097, "weighting"=w1096, "channel"=w1095, "Signal Type"=w1094) -> (w1092:T11)
      n591 = local read "Cancel"() -> (w1093:bool)
      "Canceled?" <- w1093
      n592 = for {
        tunnel: w1087 -> [w1102] mode=indexing
        tunnel: [w1101] -> w1086 mode=indexing
        n593 = Unbundle By Name(w1102) -> ("Rcv Idx"=w1101:i32)
      }
      n594 = case shown="False" w1093 {
        tunnel: w1092 -> [w1103 _]
        frame False {
          n595 = flat-sequence {
            tunnel: w1103 -> [w1104]
            frame #0 {
              n596 = global write "CRYMisc vis settings global.vi" "RTA settings"(w1104) -> ()
            }
            frame #1 {
              n597 = call "CRYSave Virtual Data.vi"() -> ()  [unwired: 1 in, 11 out]
            }
          }
        }
        frame True {
        }
      }
      n598 = call "CRYFlatten RTA.vi"("RTA settings"=w1092) -> ("Flat RTA settings"=→"RTA Setup Out":string)  [unwired: 10 out]
      n599 = Search 1D Array(1D array=w1086, element=w1085) -> (index of element=w1089:i32)  [unwired: 1 in]
      n600 = Delete From Array(array=w1087, index=w1089) -> (array with subset deleted=w1088:T23)  [unwired: 1 in, 1 out]
      n601 = global write "CRYMisc vis settings global.vi" "Rcv Index Array"(w1088) -> ()
    }
    frame #2 {
      w1113 = FALSE ("cancel")
      # "????"
      n602 = local read "Sampling rate"() -> (w1106:dbl)
      n603 = local write "Cancel"(w1113) -> ()
      n604 = local write "OK"(w1113) -> ()
      n605 = local read "dB ref."() -> (w1111:dbl)
      n606 = local read "Y Units"() -> (w1110:string)
      n607 = Bundle By Name(cluster=T4 {"Fs"=0.0, "df"=0.0, "db ref"=0.0, "X data"=1, "Y data"=0, "Y Unit"=""}, "Fs"=w1106, "df"=0.0, "db ref"=w1111, "X data"=u16 1, "Y data"=u16 0, "Y Unit"=w1110) -> (→"Data output":T4)
    }
    frame #3 {
      n608 = global read "CRYMisc vis settings global.vi" "CloseAll Event"() -> (w1117:bool)
      n609 = local read "Menu"() -> (w1115:bool)
      n610 = case shown="True" "close at end" {
        frame False {
        }
        frame True {
          n611 = property class="VI"("前面板窗口:打开"=FALSE ("Front Panel Window:Open")) -> ()  [unwired: 2 in, 2 out]
        }
      }
      n612 = Not(x=w1117) -> (.not. x?=w1116:bool)
      n613 = And(x=w1115, y=w1116) -> (x .and. y?=w1114:bool)
      n614 = case shown="True" w1114 {
        frame False {
        }
        frame True {
          n615 = local read "VI nID"() -> (w1121:i32)
          n616 = call "CRYOperator Process.vi"("VI ID"=w1121, "sAction"="Close", "sOperator Type"="OPERATOR_RTA" ("sAction")) -> ()  [unwired: 8 in, 1 out]
        }
      }
    }
    frame #4 {
      n617 = local write "StateOut"(TRUE ("StateOut")) -> ()
    }
  }
